vi "Panel.vi"(11 "StokePlot.lvlib:SinglePlotPanel.lvclass":refnum<class "RocketPlotPanel.lvclass">) -> ()   [LabVIEW 2021, in "RocketPlot.lvlib" / "RocketPlotPanel.lvclass"]
uses:
  RocketPlotPanel.lvclass
  RocketPlotPanel.lvclass/RocketPlotPanel.ctl
  <vilib>/Utility/miscctls.llb/LVPointTypeDef.ctl
  RocketPlot.lvlib
  TypeDefs/Plot UI references.ctl
  RocketPlotHandle/RocketPlotHandle.lvclass
  TypeDefs/plot while loop data.ctl
  <vilib>/Futures/Futures/Promise/Promise.lvclass
  TypeDefs/Save 1PLOT config.ctl
  RocketPlotHandle/SubVIs/Load config options.ctl
  TypeDefs/Plot general properties.ctl
  TypeDefs/Plot scale axis properties.ctl
  TypeDefs/plot attributes V2.ctl
  TypeDefs/plot properties V2.ctl
  TypeDefs/plot load data V2.ctl
  RocketPlotHandle/SubVIs/Load config.ctl
  SubVIs/CollapsePanel/CollapsePanel.lvclass
  SubVIs/CollapsePanel/SubVIs/collapse direction.ctl
  <vilib>/Utility/miscctls.llb/LVRangeTypeDef.ctl
  TypeDefs/RangeCache.ctl
  TypeDefs/MouseDownState.ctl
  <vilib>/Utility/miscctls.llb/LVPoint32TypeDef.ctl
  TypeDefs/RightClickCache.ctl
  TypeDefs/ZoomCache.ctl
  TypeDefs/RightClickCache PlatMod.ctl
  <vilib>/Utility/miscctls.llb/LVRectTypeDef.ctl
  TypeDefs/Slice average.ctl
  TypeDefs/ZoomCache PlatMod.ctl
  <userlib>/bjustice/TipStripOOPanel/Classes/TipPanelHandle/TipPanelHandle.lvclass
  <vilib>/IlluminatedG/IG OOPanel/OOPanel/Panel/Panel.lvclass
  SubVIs/Autocomplete popup/Autocomplete popup.lvlib
  SubVIs/Autocomplete popup/subvis/input options.ctl
  SubVIs/CollapsePanel/SubVIs/Expand.vi
  SubVIs/CollapsePanel/SubVIs/Collapse.vi
  SubVIs/CollapsePanel/SubVIs/Destroy.vi
  <vilib>/Utility/inputDevices.llb/closeKeyboard.vi
  TypeDefs/RightClickType.ctl
  TypeDefs/update plot queue data.ctl
  TypeDefs/plot updated return data.ctl
  TipTablePanel/TipTablePanel.lvclass
  <userlib>/bjustice/TipStripOOPanel/Classes/TipPanelHandle/CMD - shutdown.vi
  <userlib>/bjustice/TipStripOOPanel/Classes/TipPanelHandle/New.vi
  SubVIs/CollapsePanel/SubVIs/New.vi
  RocketPlotHandle/SubVIs/callback type.ctl
  RocketPlotHandle/SubVIs/callback data.ctl
  RocketPlotHandle/SubVIs/callback maximize data.ctl
  C:/Program Files/National Instruments/LabVIEW 2021/vi.lib/IlluminatedG/IG OOPanel/OOPanel/Panel/Panel.lvclass
  C:/Users/bjustice/Documents/GitHub/BluePlot/Source/Classes/RocketPlotPanel/RocketPlotPanel.lvclass
  C:/Program Files/National Instruments/LabVIEW 2021/user.lib/bjustice/TipStripOOPanel/Classes/TipPanel/TipPanel.lvclass
  C:/Users/bjustice/Documents/GitHub/BluePlot/Source/Classes/TipTablePanel/TipTablePanel.lvclass
  TypeDefs/Plot top row.ctl
  TypeDefs/TimeZone.ctl
  TypeDefs/AxisFocus.ctl
  SubVIs/menu/Plot menu activation submenu type v2.ctl
  TypeDefs/Plot axis.ctl
  TypeDefs/Shortcut Location.ctl
panel:
  in  "Plot Updated":T1
  in  "shutdown?":bool
  out "Location":T3
  out "DeferResize?":bool
  out "ShowPlotToolbar":bool
  in  "TimeZone":T6
  in  "Save 1PLOT (spoof)":bool
  in  "Load 1PLOT (spoof)":bool
  in  "Open Settings (spoof)":bool
  in  "Tab":enum32{"Page 1"}(tab)
  in  "x-axis name":string
  in  "Add row":bool
  in  "Time to Plot":dbl=1800.0 format="%<%H:%M:%S>t"
  in  "Title Visible?":bool
  in  "Erase Plot":bool
  in  "Open Settings":bool
  in  "Save 1PLOT":bool
  in  "Load 1PLOT":bool
  in  "x-axis not time?":bool caption="enable non-time x-axis?"
  in  "Scrollbar":i32(c297)
  in  "spoof1":T7(graph)
  in  "top array":T8[](array[typedef])
  in  "Title":string="Title"
  in  "PlotButtonsTab":enum32{"Page 1"}(tab)
  in  "Info":bool
  in  "max":bool
  in  "visible sidebar?":bool
  in  "Plot":cluster{dbl[], "Data":dbl[]}[](graph)
  out "RightAxisFocus":T9
  out "LeftAxisFocus":T9
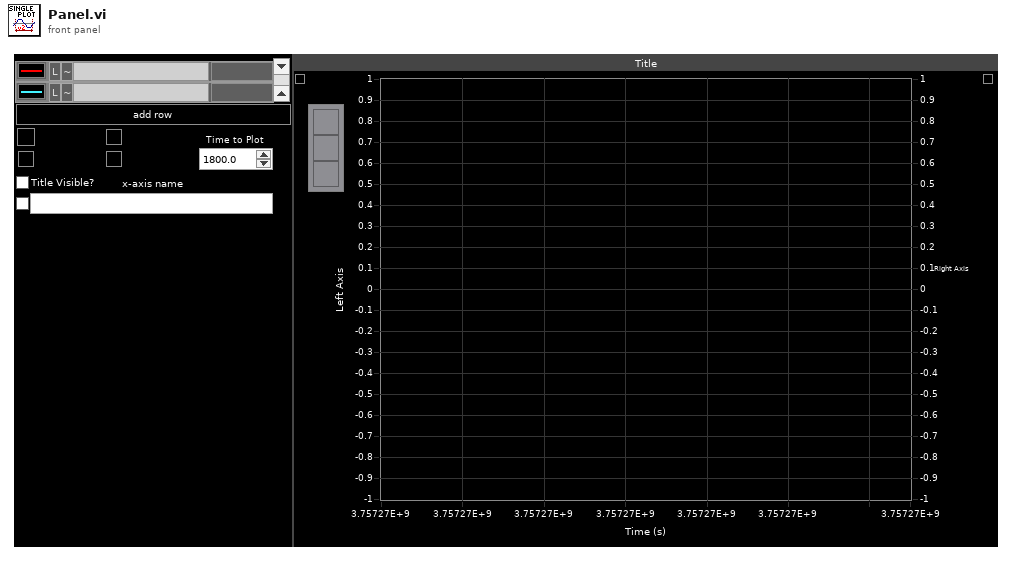
[diagram p1: front panel]
types:
  T1 = typedef "RocketPlot.lvlib/plot updated return data.ctl" = cluster{"Numerics":dbl[], "RightClickCache.slice":T2[]}
  T2 = typedef "RocketPlot.lvlib/Slice average.ctl" = cluster{"PlotIndex":i32, "Min":dbl, "Max":dbl, "Avg":dbl, "#points":u32, "Rate (Hz)":dbl, "Integral":dbl, "sigma":dbl, "CV":dbl}
  T3 = typedef "RocketPlot.lvlib/Shortcut Location.ctl" = cluster{"Location":T4, "Location.Scale":T5}
  T4 = typedef "RocketPlot.lvlib/Plot menu activation submenu type v2.ctl" = enum16{"plot area", "plot border", "markers", "scale"}
  T5 = typedef "RocketPlot.lvlib/Plot axis.ctl" = enum16{"x axis", "left axis", "right axis"}
  T6 = typedef "RocketPlot.lvlib/TimeZone.ctl" = enum16{"UTC", "Local"}
  T7 = cluster{cluster{"Time Stamp":dbl, "Data Value":dbl}[]}[]
  T8 = typedef "RocketPlot.lvlib/Plot top row.ctl" = cluster{"PID":string, "index":i32, "PID color":u32, "right axis?":bool, "Flatline?":bool, "Numeric color":u32, "Data":string, "Flat":string}
  T9 = typedef "RocketPlot.lvlib/AxisFocus.ctl" = bool
  T10 = typedef "RocketPlot.lvlib/update plot queue data.ctl" = cluster{"RightClickType":T11, "CoordsStart":T12, "CoordsEnd":T12}
  T11 = typedef "RocketPlot.lvlib/RightClickType.ctl" = enum16{"Idle", "Delta", "SliceAvg", "Identify"}
  T12 = typedef "LVPoint32TypeDef.ctl" = cluster{"Horizontal":i32, "Vertical":i32}
  T13 = typedef "CollapsePanel.lvclass/collapse direction.ctl" = enum16{"Left", "Right", "Up", "Down"}
  T14 = typedef "RocketPlot.lvlib/plot while loop data.ctl" = cluster{"TitleCollapse":refnum<class "CollapsePanel.lvclass">, "MouseDownState":T15, "RightClickCache":T16, "ZoomCache":T19, "UpdateTime":dbl, "keyboard":refnum<k1>, "visible?":bool}
  T15 = typedef "RocketPlot.lvlib/MouseDownState.ctl" = enum16{"Idle", "Pan", "Zoom", "Zoom-Post", "RightClick"}
  T16 = typedef "RocketPlot.lvlib/RightClickCache.ctl" = cluster{"Mod":T17, "CoordsStart":T12, "CoordsEnd":T12, "PlotAreaBounds":T18, "slice":T2[]}
  T17 = typedef "RocketPlot.lvlib/RightClickCache PlatMod.ctl" = cluster{"Ctrl":bool, "Shift":bool}
  T18 = typedef "LVRectTypeDef.ctl" = cluster{"Left":i16, "Top":i16, "Right":i16, "Bottom":i16}
  T19 = typedef "RocketPlot.lvlib/ZoomCache.ctl" = cluster{"SuppressedPlots":i32[], "LeftAxis":T20, "RightAxis":T20, "Mod":T22}
  T20 = typedef "RocketPlot.lvlib/RangeCache.ctl" = cluster{"NeedsRevert?":bool, "Scale Fit":u8, "Range":T21}
  T21 = typedef "LVRangeTypeDef.ctl" = cluster{"Minimum":dbl, "Maximum":dbl, "Increment":dbl, "Minor Increment":dbl, "Start":dbl}
  T22 = typedef "RocketPlot.lvlib/ZoomCache PlatMod.ctl" = cluster{"Shift":bool}
  T23 = typedef "RocketPlot.lvlib/Plot UI references.ctl" = cluster{"Title":refnum<vi>, "Title?":refnum<vi>, "Visible sidebar?":refnum<vi>, "Time to Plot":refnum<vi>, "top array":refnum<vi>, "Scrollbar":refnum<vi>, "tab ref":refnum<vi>, "Add row":refnum<vi>, "TopArray":cluster{"PID":refnum<vi>, "Numeric color":refnum<vi>, "Flat":refnum<vi>, "PID color":refnum<vi>, "Data":refnum<vi>}, "Splitter":refnum<vi>, "Front Panel":refnum<vi>, "VI":refnum<vi>, "Meta LUT":refnum<data-value>, "spoof":refnum<vi>, "BluePlotHandle":refnum<class "RocketPlotHandle.lvclass">, "PlotPane":refnum<vi>, "X Scale":refnum<vi>, "Left Scale":refnum<vi>, "Right Scale":refnum<vi>, "TimeZone":refnum<vi>, "ShowPlotToolBar":refnum<vi>, "DeferResize?":refnum<vi>, "LegendPane":refnum<vi>, "Plot":refnum<vi>, "PlotToolBar":refnum<vi>, "TB.Info":refnum<vi>, "TB.max":refnum<vi>, "X Scale.Plot Name":refnum<vi>, "X Scale.Use Plot Name?":refnum<vi>, "TipPanel":refnum<class "TipPanelHandle.lvclass">}
  T24 = typedef "RocketPlotHandle.lvclass/Init Options.ctl" = cluster{"UI visible?":bool, "Update rate (ms)":u32, "Sidebar.Visible":bool, "time to plot (init)":dbl, "time to plot (max)":dbl, "config file start path":path, "Title.Visible":bool, "Title":string, "TimeZone":T6}
  T25 = typedef "LVPointTypeDef.ctl" = cluster{"Horizontal":i16, "Vertical":i16}
  T26 = typedef "OOPanel.lvlib/Panel.lvclass/Panel Events.ctl" = cluster{"Visbility":refnum<user-event>, "Close":refnum<user-event>}
  T27 = typedef "RocketPlot.lvlib/panel mode.ctl" = enum16{"1PLOT", "MPLOT"}
  T28 = typedef "RocketPlotHandle.lvclass/callback type.ctl" = enum16{"Maximize", "ShortcutMenu"}
  T29 = typedef "RocketPlotHandle.lvclass/callback data.ctl" = cluster{"Type":T28, "data":variant, "owning subpanel":refnum<vi>}
  T30 = typedef "RocketPlot.lvlib/Save 1PLOT config.ctl" = cluster{"file extension":string, "start path":path}
  T31 = typedef "RocketPlotHandle.lvclass/Load config options.ctl" = cluster{"Load plots?":bool, "Load X-axis?":bool, "Load Y-axes?":bool, "Load General?":bool}
  T32 = typedef "RocketPlotHandle.lvclass/Load config.ctl" = cluster{"Plot config":T33, "Load options (All)":T31}
  T33 = typedef "RocketPlot.lvlib/plot load data V2.ctl" = cluster{"plots":T34[], "X-axis":T36, "Y-axes":T36[], "General":T37}
  T34 = typedef "RocketPlot.lvlib/plot properties V2.ctl" = cluster{"attributes":T35, "Numeric":dbl, "Flatline?":bool}
  T35 = typedef "RocketPlot.lvlib/plot attributes V2.ctl" = cluster{"Plot Color":u32, "Point Style":u8, "Line Style":u8, "Plot Interpolation":u8, "Line Width":u8, "Bar Plot Style":u8, "Fill To":i16, "X Scale Index":u32, "Y Scale Index":u32, "Anti-aliased":bool, "Label Format":u8, "Digital Transition Type":u8, "Digital Transition Location":u8, "Digital Line Style":u8, "Fill/Point Color":u32, "Plot Name":string, "Visible":bool}
  T36 = typedef "RocketPlot.lvlib/Plot scale axis properties.ctl" = cluster{"Name Label.Text":string, "Style":u8, "Tick Colors:Minor Tick Color":u32, "Tick Colors:Tick Color":u32, "Marker Colors:Text Color":u32, "Grid Colors:Major Color":u32, "Grid Colors:Minor Color":u32, "Mapping Mode":u8, "Flipped":bool, "Name Label.Visible":bool, "Name Label.Text Colors:Text Color":u32, "Scale Fit":u8, "Range:Maximum":dbl, "Range:Minimum":dbl, "Offset and Multiplier:Multiplier":dbl, "Offset and Multiplier:Offset":dbl, "Name Label.Font:Size":u32, "Marker.Font:Size":u32, "Uniform Marker Spacing?":bool, "Format String":string}
  T37 = typedef "RocketPlot.lvlib/Plot general properties.ctl" = cluster{"Title":string, "Time to Plot":dbl, "Title.Visible":bool, "Sidebar.Visible":bool, "Plot Area:Colors:BG Color":u32, "X Scale.Plot Name":string, "X Scale.Use Plot Name":bool}
  T38 = typedef "RocketPlotHandle.lvclass/callback maximize data.ctl" = cluster{"Maximize?":bool, "max button":refnum<vi>}
  T39 = typedef "Autocomplete popup.lvlib/input options.ctl" = cluster{"Screen Coordinates":T25, "Width":u32, "max rows":i32, "List":string[], "init value":string}
  T40 = cluster{"Color":u32, "PointStyle":u8, "LineStyle":u8, "Interp":u8, "LineWidth":u8, "BarPlotStyle":u8, "FillTo":i16, "XScaleIdx":u32, "YScaleIdx":u32, "Anti-Aliased":bool, "LabelFormat":u8, "TransitionType":u8, "TransitionLocation":u8, "DigitalLineStyle":u8}
  T41 = typedef "Plot top row.ctl" = cluster{"PID":string, "index":i32, "PID color":u32, "right axis?":bool, "Flatline?":bool, "Numeric color":u32, "Data":string, "Flat":string}
  T42 = typedef "RocketPlot.lvlib/TipTablePanel.lvclass/cell cache.ctl" = cluster{"text":string, "Color":u32, "Justification":enum16{"Left", "Center", "Right"}}
  T43 = typedef "StokePlot.lvlib/Plot QSM action.ctl" = enum16{"Get Config", "Load Config", "Set TimeToPlot", "Clear Config"}
  T44 = typedef "OOPanel.lvlib/Visibility State.ctl" = enum16{"Idle", "Closed", "Hidden", "Visible", "Subpanel", "Hidden Subpanel"}
  T45 = cluster{"Shift":bool, "Ctrl":bool, "Alt":bool, "Cmd":bool, "Opt":bool}
  T46 = typedef "eventvkey.ctl" = enum16{"ASCII", "Enter", "Return", "Shift", "Ctrl", "Alt", "Cmd", "Opt", "Caps", "NumLock", "Clear", "Break", "Up", "Down", "Left", "Right", "Insert", "Delete", "Home", "End", "PageUp", "PageDown", "Escape", "Help", "Pause", "ScrollLock", "F1", "F2", "F3", "F4", "F5", "F6", "F7", "F8", "F9", "F10", "F11", "F12", "F13", "F14", "F15", "F16", "F17", "F18", "F19", "F20", "F21", "F22", "F23", "F24", "Play", "VolumeUp", "VolumeDown", "Mute", "Two Byte Char"}
  T47 = typedef "RocketPlot.lvlib/Plot scale meta JSON.ctl" = cluster{"Type":T5, "Grid Colors:Major Color":u32, "Grid Colors:Minor Color":u32, "Style":u8, "Tick Colors:Tick Color":u32, "Tick Colors:Minor Tick Color":u32, "Format String":string, "State":T48, "AxisFocus":refnum<vi>}
  T48 = typedef "RocketPlot.lvlib/Plot scale meta state.ctl" = cluster{"Visible":bool, "Focus":bool, "Multi-Y":bool}
  T49 = typedef "TimeZone.ctl" = enum16{"UTC", "Local"}
  T50 = typedef "LVPositionTypeDef.ctl" = cluster{"Left":i32, "Top":i32}
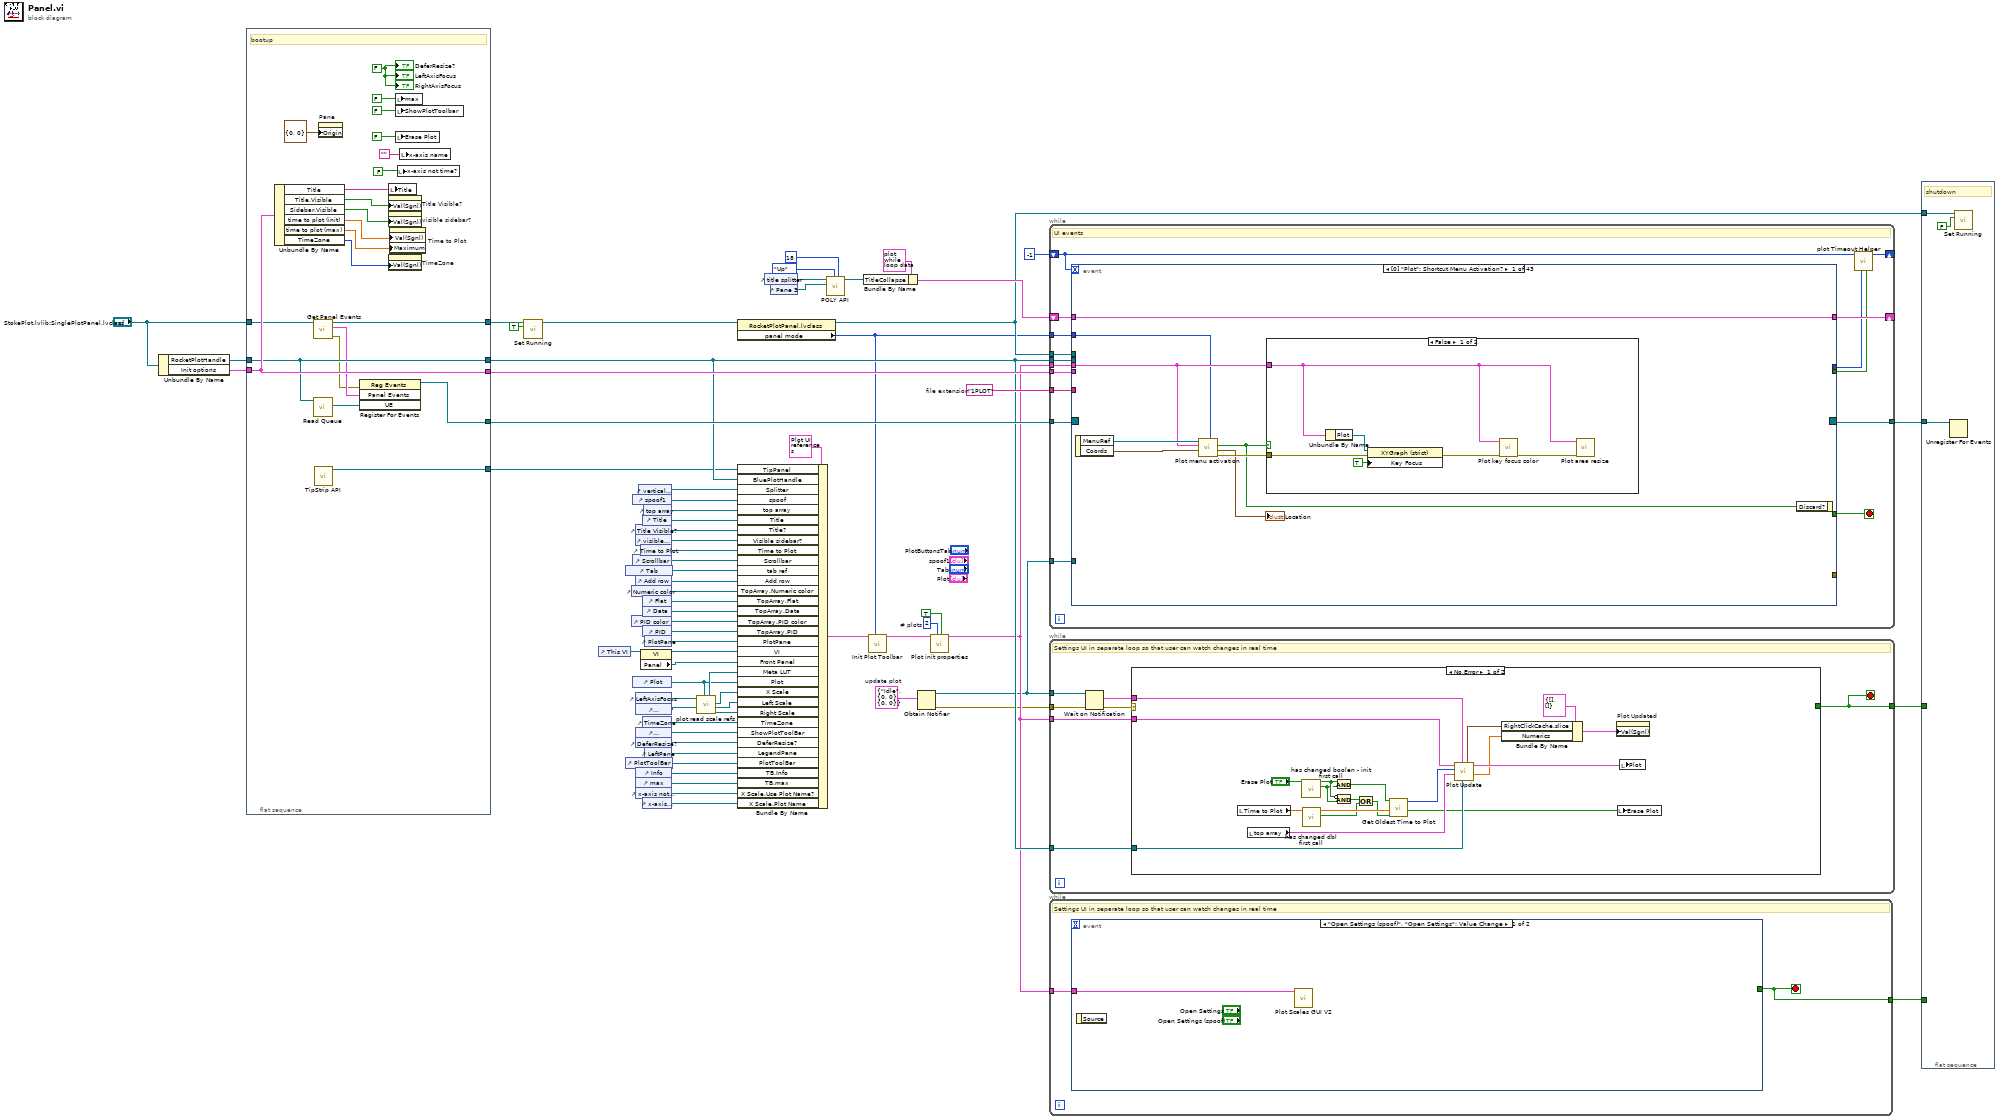
[diagram p0: block diagram]
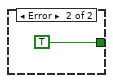
[diagram p2: hidden frame]
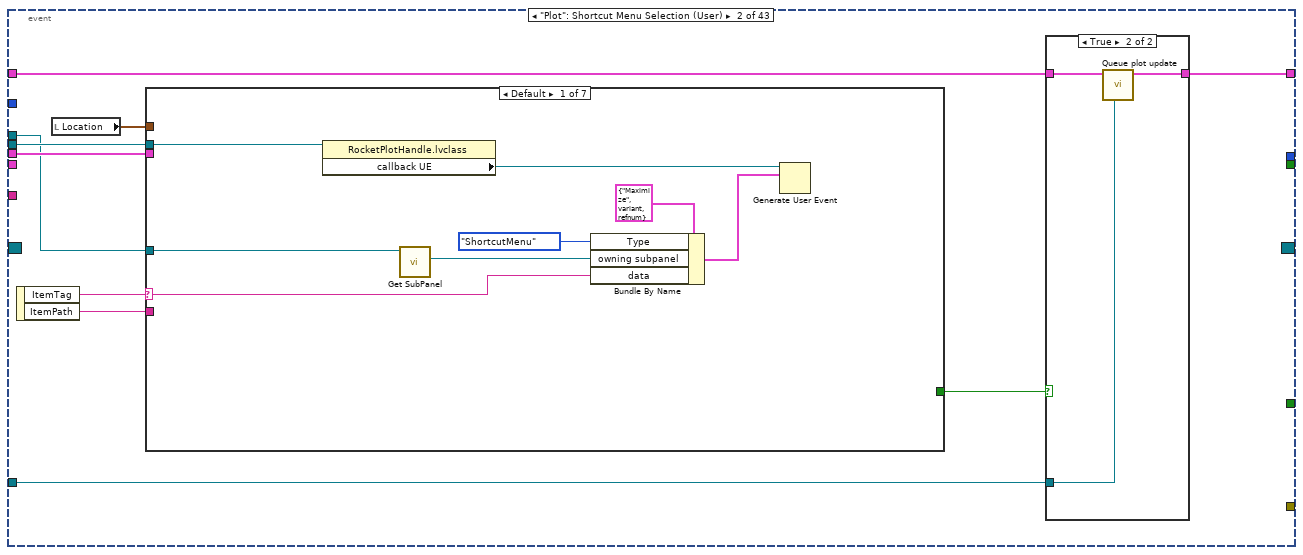
[diagram p4: hidden frame]
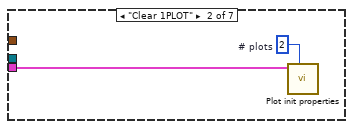
[diagram p6: hidden frame]
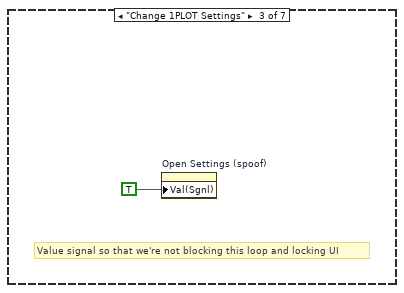
[diagram p7: hidden frame]
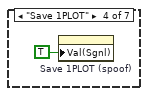
[diagram p8: hidden frame]
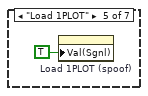
[diagram p9: hidden frame]
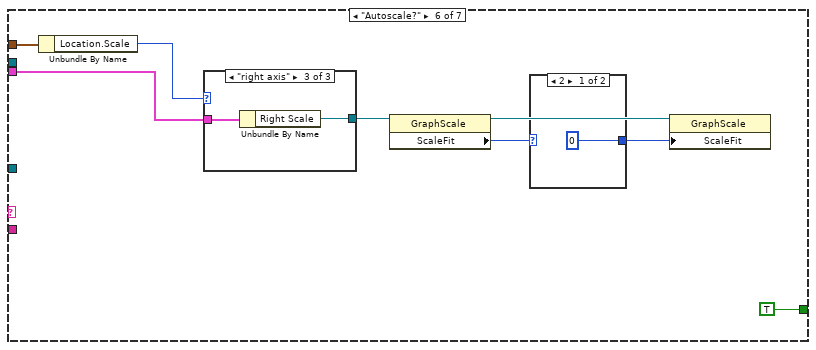
[diagram p10: hidden frame]
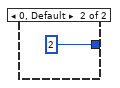
[diagram p11: hidden frame]
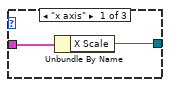
[diagram p12: hidden frame]
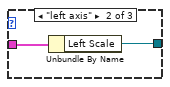
[diagram p13: hidden frame]
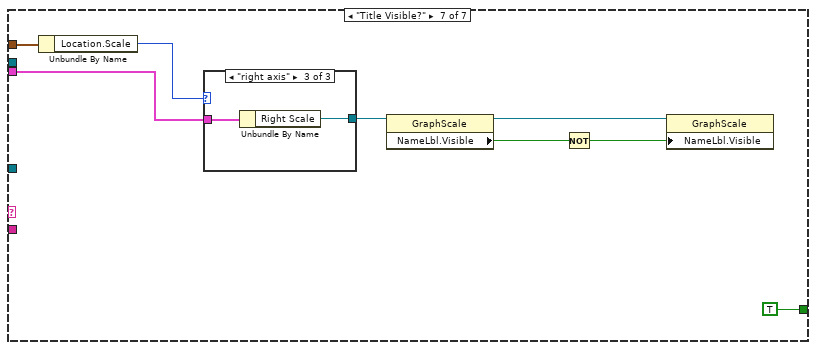
[diagram p14: hidden frame]
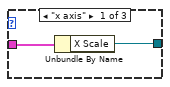
[diagram p15: hidden frame]
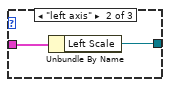
[diagram p16: hidden frame]
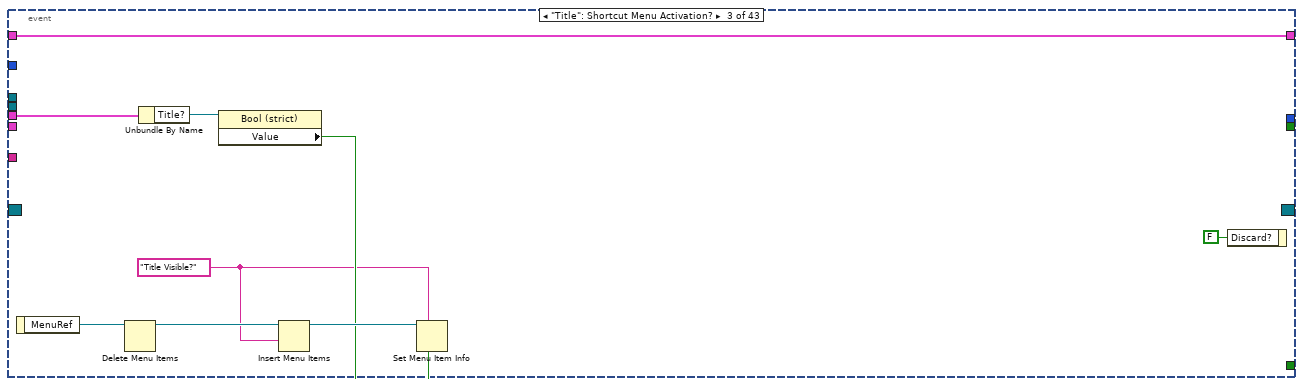
[diagram p17: hidden frame]
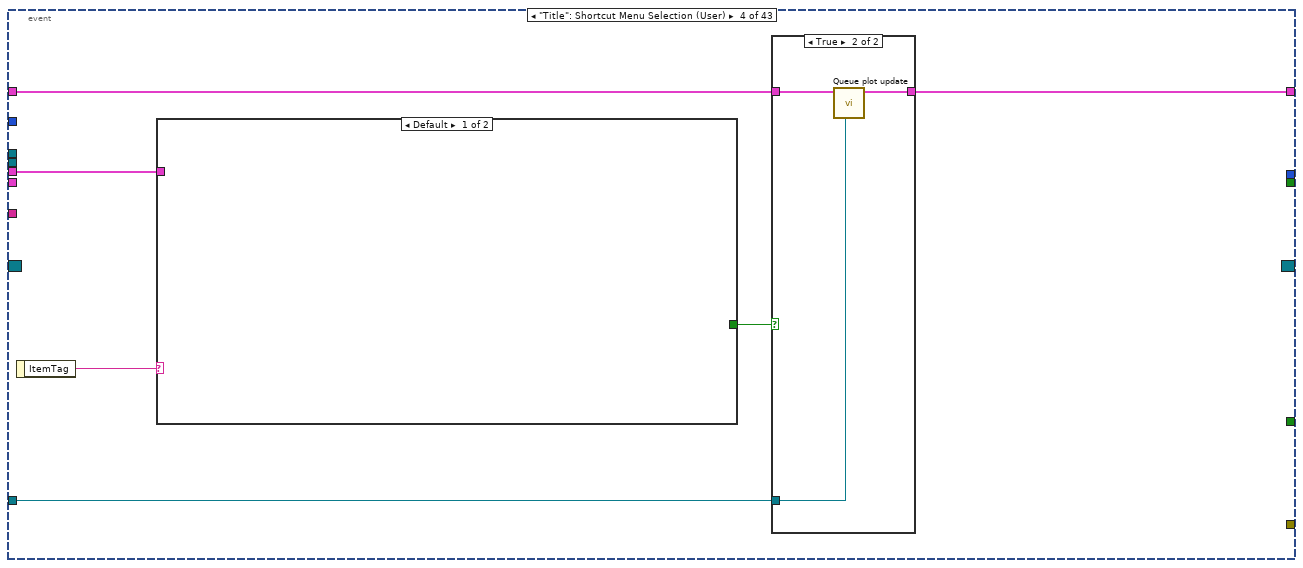
[diagram p18: hidden frame]
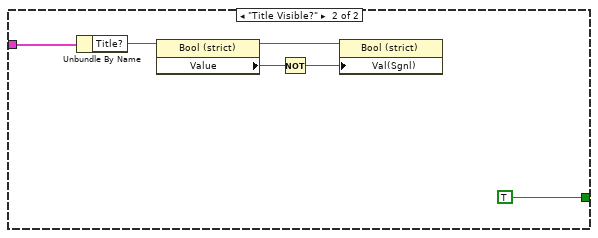
[diagram p20: hidden frame]
diagram:
  w7 = T10 {"RightClickType"=enum."Idle", "CoordsStart"={"Horizontal"=0, "Vertical"=0}, "CoordsEnd"={"Horizontal"=0, "Vertical"=0}}  # update plot
  w49 = "1PLOT"  # file extension
  w62 = 2  # # plots
  n1 = Unbundle By Name("StokePlot.lvlib:SinglePlotPanel.lvclass") -> ("RocketPlotHandle"=w17:refnum<class "RocketPlotHandle.lvclass">, "Init options"=w18:T24)
  n2 = flat-sequence {
    tunnel: [w90] -> w47
    tunnel: [w83] -> w9
    tunnel: w17 -> [w83]
    tunnel: w18 -> [w84]
    tunnel: [w84] -> w46
    tunnel: "StokePlot.lvlib:SinglePlotPanel.lvclass" -> [w76]
    tunnel: [w72] -> w15
    tunnel: [w70] -> w4
    frame #0 {
      w78 = FALSE ("DeferResize?")
      # "bootup"
      n3 = Unbundle By Name(w84) -> ("Title"=w89:string, "Title.Visible"=w88:bool, "Sidebar.Visible"=w80:bool, "time to plot (init)"=w86:dbl, "time to plot (max)"=w87:dbl, "TimeZone"=w69:T6)
      n4 = call <vilib>:"Get Panel Events.vi"("Panel in"=w76) -> ("error out"=w74:errorcluster, "Panel Events"=w75:T26, "Panel out"=w72:refnum<class "RocketPlotPanel.lvclass">)  [unwired: 8 in]
      n5 = call "Read Queue.vi"("BluePlotHandle in"=w83) -> ("UE"=w77:refnum<user-event>)  [unwired: 8 in, 2 out]
      n6 = call-poly <userlib>:"TipStrip API.vi"() -> ("TipPanelHandle out"=w70:refnum<class "TipPanelHandle.lvclass">)  [unwired: 10 in, 1 out]
      n7 = property on="Pane" class="Pane"("Origin"=T25 {"Horizontal"=0, "Vertical"=0}) -> ()  [unwired: 2 in, 2 out]
      n8 = register-events(error in=w74, w75, w77) -> (reference out=w90:refnum<event-registration>)  [unwired: 1 in, 1 out]
      n9 = local write "Title"(w89) -> ()
      n10 = property on="Title Visible?" class="Bool (strict)"("Val(Sgnl)"=w88) -> ()  [unwired: 2 in, 2 out]
      n11 = property on="visible sidebar?" class="Bool (strict)"("Val(Sgnl)"=w80) -> ()  [unwired: 2 in, 2 out]
      n12 = property on="TimeZone" class="Enum (strict)"("Val(Sgnl)"=w69) -> ()  [unwired: 2 in, 2 out]
      n13 = property on="Time to Plot" class="DigNum (strict)"("Val(Sgnl)"=w86, "Maximum"=w87) -> ()  [unwired: 2 in, 2 out]
      n14 = local write "max"(FALSE ("max")) -> ()
      n15 = local write "ShowPlotToolbar"(FALSE ("ShowCollapseButton")) -> ()
      n16 = local write "Erase Plot"(FALSE ("Clear Plots")) -> ()
      n17 = local write "x-axis not time?"(FALSE ("Value (Signaling)")) -> ()
      n18 = local write "x-axis name"("") -> ()
      "LeftAxisFocus" <- w78
      "RightAxisFocus" <- w78
      "DeferResize?" <- w78
    }
  }
  n19 = call <vilib>:"Set Running.vi"("Running"=TRUE, "Panel in"=w15) -> ("Panel out"=w3:refnum<class "RocketPlotPanel.lvclass">)  [unwired: 8 in, 1 out]
  n20 = control-ref of="This VI"() -> (w58:refnum<vi>)
  n21 = control-ref of="Tab"() -> (w63:refnum<vi>)
  n22 = control-ref of="PlotToolBar"() -> (w24:refnum<vi>)
  n23 = control-ref of="Numeric color"() -> (w53:refnum<vi>)
  n24 = control-ref of="PID color"() -> (w50:refnum<vi>)
  n25 = control-ref of="spoof1"() -> (w61:refnum<vi>)
  n26 = control-ref of="Scrollbar"() -> (w64:refnum<vi>)
  n27 = control-ref of="Plot"() -> (w26:refnum<vi>)
  n28 = control-ref of="Title Visible?"() -> (w66:refnum<vi>)
  n29 = control-ref of="visible sidebar?"() -> (w25:refnum<vi>)
  n30 = control-ref of="Add row"() -> (w59:refnum<vi>)
  n31 = control-ref of="LeftAxisFocus"() -> (w37:refnum<vi>)
  n32 = control-ref of="RightAxisFocus"() -> (w36:refnum<vi>)
  n33 = control-ref of="ShowPlotToolbar"() -> (w38:refnum<vi>)
  n34 = control-ref of="DeferResize?"() -> (w28:refnum<vi>)
  n35 = control-ref of="Info"() -> (w23:refnum<vi>)
  n36 = control-ref of="max"() -> (w22:refnum<vi>)
  n37 = control-ref of="x-axis not time?"() -> (w14:refnum<vi>)
  n38 = control-ref of="vertical splitter"() -> (w57:refnum<vi>)
  n39 = control-ref of="Time to Plot"() -> (w67:refnum<vi>)
  n40 = property class="VI"(reference=w58) -> (reference out=w55:refnum<vi>, "Panel"=w56:refnum<vi>)  [unwired: 1 in, 1 out]
  n41 = control-ref of="Title"() -> (w65:refnum<vi>)
  n42 = control-ref of="Flat"() -> (w52:refnum<vi>)
  n43 = control-ref of="Data"() -> (w51:refnum<vi>)
  n44 = control-ref of="PID"() -> (w54:refnum<vi>)
  n45 = control-ref of="TimeZone"() -> (w40:refnum<vi>)
  n46 = control-ref of="x-axis name"() -> (w11:refnum<vi>)
  n47 = control-ref of="top array"() -> (w60:refnum<vi>)
  n48 = control-ref of="PlotPane"() -> (w48:refnum<vi>)
  n49 = control-ref of="LeftPane"() -> (w27:refnum<vi>)
  n50 = call "plot read scale refs.vi"("Plot"=w26, "RightAxisFocus"=w36, "LeftAxisFocus"=w37) -> ("Right Scale"=w43:refnum<vi>, "Left Scale"=w42:refnum<vi>, "X Scale"=w41:refnum<vi>, "Meta LUT"=w39:refnum<data-value>)  [unwired: 4 in, 1 out]
  n51 = property class="RocketPlotPanel.lvclass"(reference=w3) -> (reference out=w2:refnum<class "RocketPlotPanel.lvclass">, "panel mode"=w1:T27)  [unwired: 1 in, 1 out]
  n52 = Bundle By Name(cluster=T23 {"Title"=refnum, "Title?"=refnum, "Visible sidebar?"=refnum, "Time to Plot"=refnum, "top array"=refnum, "Scrollbar"=refnum, "tab ref"=refnum, "Add row"=refnum, "TopArray"={"PID"=refnum, "Numeric color"=refnum, "Flat"=refnum, "PID color"=refnum, "Data"=refnum}, "Splitter"=refnum, "Front Panel"=refnum, "VI"=refnum, "Meta LUT"=refnum, "spoof"=refnum, "BluePlotHandle"=refnum, "PlotPane"=refnum, "X Scale"=refnum, "Left Scale"=refnum, "Right Scale"=refnum, "TimeZone"=refnum, "ShowPlotToolBar"=refnum, "DeferResize?"=refnum, "LegendPane"=refnum, "Plot"=refnum, "PlotToolBar"=refnum, "TB.Info"=refnum, "TB.max"=refnum, "X Scale.Plot Name"=refnum, "X Scale.Use Plot Name?"=refnum, "TipPanel"=refnum} ("Cluster"), "TipPanel"=w4, "BluePlotHandle"=w9, "Splitter"=w57, "spoof"=w61, "top array"=w60, "Title"=w65, "Title?"=w66, "Visible sidebar?"=w25, "Time to Plot"=w67, "Scrollbar"=w64, "tab ref"=w63, "Add row"=w59, "TopArray.Numeric color"=w53, "TopArray.Flat"=w52, "TopArray.Data"=w51, "TopArray.PID color"=w50, "TopArray.PID"=w54, "PlotPane"=w48, "VI"=w55, "Front Panel"=w56, "Meta LUT"=w39, "Plot"=w26, "X Scale"=w41, "Left Scale"=w42, "Right Scale"=w43, "TimeZone"=w40, "ShowPlotToolBar"=w38, "DeferResize?"=w28, "LegendPane"=w27, "PlotToolBar"=w24, "TB.Info"=w23, "TB.max"=w22, "X Scale.Use Plot Name?"=w14, "X Scale.Plot Name"=w11) -> (w21:T23)
  n53 = control-ref of="title splitter"() -> (w33:refnum<vi>)
  n54 = control-ref of="Pane 3"() -> (w32:refnum<vi>)
  n55 = call-poly "POLY API.vi"("ExpandSize (starting size)"=18, "CollapseDirection"=collapse_direction."Up", "Pane"=w32, "Splitter"=w33) -> ("CollapsePanel out"=w30:refnum<class "CollapsePanel.lvclass">)  [unwired: 6 in, 1 out]
  n56 = Bundle By Name(cluster=T14 {"TitleCollapse"=refnum, "MouseDownState"=enum."Idle", "RightClickCache"={"Mod"={"Ctrl"=FALSE, "Shift"=FALSE}, "CoordsStart"={"Horizontal"=0, "Vertical"=0}, "CoordsEnd"={"Horizontal"=0, "Vertical"=0}, "PlotAreaBounds"={"Left"=10, "Top"=10, "Right"=0, "Bottom"=0}, "slice"=[]}, "ZoomCache"={"SuppressedPlots"=[], "LeftAxis"={"NeedsRevert?"=FALSE, "Scale Fit"=0, "Range"={"Minimum"=0.0, "Maximum"=0.0, "Increment"=0.0, "Minor Increment"=0.0, "Start"=0.0}}, "RightAxis"={"NeedsRevert?"=FALSE, "Scale Fit"=0, "Range"={"Minimum"=0.0, "Maximum"=0.0, "Increment"=0.0, "Minor Increment"=0.0, "Start"=0.0}}, "Mod"={"Shift"=FALSE}}, "UpdateTime"=0.0, "keyboard"=refnum, "visible?"=FALSE} ("loop data"), "TitleCollapse"=w30) -> (w29:T14)
  n57 = call "Init Plot Toolbar.vi"("panel mode"=w1, "Refs"=w21) -> ("Refs (dup)"=w20:T23)  [unwired: 8 in, 1 out]
  n58 = Obtain Notifier(notification data type=w7) -> (notifier out=w6:refnum<notifier>, error out=w5:errorcluster)  [unwired: 3 in, 1 out]
  n59 = call "Plot init properties.vi"("First call? (init)"=TRUE, "# plots"=w62, "Refs"=w20) -> ("Refs (dup)"=w8:T23)  [unwired: 7 in, 1 out]
  n60 = while {
    tunnel: w8 -> [w106]
    tunnel: w9 -> [w105]
    tunnel: w46 -> [w104]
    tunnel: w49 -> [w103]
    tunnel: w47 -> [w102]
    shift-right: [w97] -> _
    shift-left: -1 ("Timeout") -> [w96]
    tunnel: [w100] -> w45
    shift-right: [w98] -> _
    shift-left: w29 -> [w99]
    tunnel: w6 -> [w93]
    tunnel: w2 -> [w92]
    tunnel: w1 -> [w91]
    stop <- w101 stop-if-true
    # "UI events"
    n61 = event shown="[0] \"Plot\": Shortcut Menu Activation?" {
      selector: w102 -> [_ _ _ _ _ _ _ _ _ _ _ _ _ _ _ _ _ _ _ _ _ _ _ _ _ _ _ _ _ _ _ _ _ _ _ _ _ _ _ _ _ _ _]
      dyn-events: [_ _ _ _ _ _ _ _ _ _ _ _ _ _ _ _ _ _ _ _ _ _ _ _ _ _ _ _ _ _ _ _ _ _ _ _ _ _ _ _ _ _ _] -> w100
      timeout: w96 -> [_ _ _ _ _ _ _ _ _ _ _ _ _ _ _ _ _ _ _ _ _ _ _ _ _ _ _ _ _ _ _ _ _ _ _ _ _ _ _ _ _ _ _]
      tunnel: [_ _ _ _ w209 w218 _ w230 w239 w252 w265 w282 _ _ _ w305 _ _ w320 _ _ _ _ _ _ _ _ _ _ _ _ _ _ _ _ _ _ _ _ _ _ _ _] -> _
      tunnel: w106 -> [w112 w127 w183 w191 w210 w211 _ w229 w238 w251 _ w277 w291 w299 _ w306 w311 w316 w324 w329 _ w377 w386 w404 w424 w439 w468 w484 w492 w505 w529 w548 w554 w560 w564 w579 w584 w595 w610 w630 w657 w670 w674]
      tunnel: w105 -> [_ w129 _ _ _ _ _ _ _ _ _ _ _ _ w303 _ _ _ _ w328 _ w372 _ _ _ _ _ _ _ _ _ _ _ _ _ w569 _ _ _ w631 w654 _ _]
      tunnel: w104 -> [_ _ _ _ w207 w215 _ _ _ _ _ _ _ _ _ _ _ _ _ w325 w365 _ w389 _ w423 _ w473 w481 _ w499 w524 _ _ _ _ _ _ _ _ _ _ _ _]
      tunnel: w103 -> [_ _ _ _ w204 w213 _ _ _ _ _ _ _ _ _ _ _ _ _ _ _ _ _ _ _ _ _ _ _ _ _ _ _ _ _ _ _ _ _ _ _ _ _]
      tunnel: [_ _ _ _ _ _ _ _ _ _ _ _ _ _ _ _ _ _ _ _ w366 _ w387 _ w421 _ _ w482 _ _ _ _ _ _ _ _ _ _ _ _ _ _ _] -> w95
      tunnel: [_ _ _ _ _ _ _ _ _ _ _ _ _ _ _ _ _ _ _ _ w367 _ w388 _ w422 _ _ w483 _ _ _ _ _ _ _ _ _ _ _ _ _ _ _] -> w94
      tunnel: [_ _ _ _ _ _ _ _ _ _ _ _ _ _ _ _ _ _ _ _ _ w376 _ _ _ _ _ _ _ _ _ _ _ _ _ _ _ _ _ _ _ _ _] -> w101
      tunnel: w99 -> [w113 w124 w178 w189 w203 w212 w224 w226 w237 w250 w264 w283 w292 w300 w301 w304 w309 w314 w323 w327 w369 w378 w391 w407 w425 w441 w470 w485 w491 w504 w528 w547 w558 w562 w567 w580 w590 w596 w599 w632 w655 w669 w673]
      tunnel: [w113 w123 w178 w188 w203 w212 w224 w226 w237 w250 w263 w283 w292 w300 w301 w304 w309 w314 w323 w326 w368 w378 w384 w408 w420 w441 w466 w479 w487 w494 w519 w542 w558 w562 w567 w580 w590 w596 w598 w632 w655 w669 w673] -> w98
      tunnel: w93 -> [_ w122 _ w187 _ _ _ _ _ _ _ _ _ _ _ _ _ _ _ _ _ w375 w383 _ _ _ w465 w478 w486 w493 w518 w540 _ _ _ _ _ _ w597 _ _ _ _]
      tunnel: w92 -> [_ w121 _ _ _ _ _ _ _ _ _ _ _ _ _ _ _ _ _ _ _ _ _ _ _ _ _ _ _ _ _ _ _ _ _ w570 _ _ _ _ _ _ _]
      tunnel: w91 -> [w107 _ _ _ _ _ _ _ _ _ _ _ _ _ _ _ _ _ _ _ _ _ _ _ _ _ _ _ _ _ _ _ _ _ _ _ _ _ _ _ _ _ _]
      event "Plot": Shortcut Menu Activation? {
        n62 = event-data() -> ("MenuRef"=w114:refnum<k9>, "Coords"=w111:T12)  [unwired: 1 in]
        n63 = call "Plot menu activation.vi"("panel mode"=w107, "Coords"=w111, "Refs"=w112, "MenuRef"=w114) -> ("error out"=w110:errorcluster, "Location"=→"Location":T3, "Discard?"=w108:bool)  [unwired: 4 in, 1 out]
        n64 = case shown="False" w108 {
          tunnel: w112 -> [w120 _]
          tunnel: w110 -> [w118 _]
          frame False {
            n65 = Unbundle By Name(w120) -> ("Plot"=w117:refnum<vi>)
            n66 = property class="XYGraph (strict)"(reference=w117, error in=w118, "Key Focus"=TRUE) -> (error out=w115:errorcluster)  [unwired: 1 out]
            n67 = call "Plot key focus color.vi"("error in (no error)"=w115, "Refs"=w120) -> ("error out"=w116:errorcluster)  [unwired: 9 in]
            n68 = call "Plot area resize.vi"("error in (no error)"=w116, "Refs"=w120) -> ()  [unwired: 9 in, 1 out]
          }
          frame True {
          }
        }
        n69 = event-data("Discard?"=w108) -> ()  [unwired: 1 in, 1 out]
      }
      event "Plot": Shortcut Menu Selection (User) {
        n70 = event-data() -> ("ItemTag"=w130:string, "ItemPath"=w128:string)  [unwired: 1 in]
        n71 = local read "Location"() -> (w126:T3)
        n72 = case shown="Default" w130 {
          selector: w130 -> [w137 _ _ _ _ _ _]
          tunnel: w129 -> [w136 _ _ _ _ _ _]
          tunnel: w128 -> [_ _ _ _ _ _ _]
          tunnel: w127 -> [_ w143 _ _ _ w153 w169]
          tunnel: w126 -> [_ _ _ _ _ w154 w170]
          tunnel: [_ _ _ _ _ TRUE TRUE] -> w125
          tunnel: w121 -> [w135 _ _ _ _ _ _]
          frame Default {
            n73 = property class="RocketPlotHandle.lvclass"(reference=w136) -> ("callback UE"=w138:refnum<user-event>)  [unwired: 1 in, 2 out]
            n74 = call <vilib>:"Get SubPanel.vi"("Panel in"=w135) -> ("SubPanel"=w139:refnum<vi>)  [unwired: 8 in, 2 out]
            n75 = Bundle By Name(cluster=T29 {"Type"=enum."Maximize", "data"=variant(string ""), "owning subpanel"=refnum} ("event data"), "Type"=callback_type."ShortcutMenu", "owning subpanel"=w139, "data"=w137) -> (w141:T29)
            n76 = Generate User Event(user event=w138, event data cluster=w141) -> ()  [unwired: 2 in, 2 out]
          }
          frame "Clear 1PLOT" {
            w144 = 2  # # plots
            n77 = call "Plot init properties.vi"("# plots"=w144, "Refs"=w143) -> ()  [unwired: 8 in, 2 out]
          }
          frame "Change 1PLOT Settings" {
            # "Value signal so that we're not blocking this loop and locking UI"
            n78 = property on="Open Settings (spoof)" class="Bool (strict)"("Val(Sgnl)"=TRUE ("Value (Signaling)")) -> ()  [unwired: 2 in, 2 out]
          }
          frame "Save 1PLOT" {
            n79 = property on="Save 1PLOT (spoof)" class="Bool (strict)"("Val(Sgnl)"=TRUE ("Value (Signaling)")) -> ()  [unwired: 2 in, 2 out]
          }
          frame "Load 1PLOT" {
            n80 = property on="Load 1PLOT (spoof)" class="Bool (strict)"("Val(Sgnl)"=TRUE ("Value (Signaling)")) -> ()  [unwired: 2 in, 2 out]
          }
          frame "Autoscale?" {
            n81 = Unbundle By Name(w154) -> ("Location.Scale"=w152:T5)
            n82 = case shown="\"right axis\"" w152 {
              tunnel: w153 -> [w159 w161 w163]
              tunnel: [w158 w160 w162] -> w155
              frame "x axis" {
                n83 = Unbundle By Name(w159) -> ("X Scale"=w158:refnum<vi>)
              }
              frame "left axis" {
                n84 = Unbundle By Name(w161) -> ("Left Scale"=w160:refnum<vi>)
              }
              frame "right axis" {
                n85 = Unbundle By Name(w163) -> ("Right Scale"=w162:refnum<vi>)
              }
            }
            n86 = property class="GraphScale"(reference=w155) -> (reference out=w151:refnum<vi>, "ScaleFit"=w150:u8)  [unwired: 1 in, 1 out]
            n87 = case shown="2" w150 {
              tunnel: [u8 0 ("Scale Fit") u8 2 ("Scale Fit")] -> w149
              frame 2 {
              }
              frame 0, Default {
              }
            }
            n88 = property class="GraphScale"(reference=w151, "ScaleFit"=w149) -> ()  [unwired: 1 in, 2 out]
          }
          frame "Title Visible?" {
            n89 = Unbundle By Name(w170) -> ("Location.Scale"=w168:T5)
            n90 = case shown="\"right axis\"" w168 {
              tunnel: w169 -> [w173 w175 w177]
              tunnel: [w172 w174 w176] -> w171
              frame "x axis" {
                n91 = Unbundle By Name(w173) -> ("X Scale"=w172:refnum<vi>)
              }
              frame "left axis" {
                n92 = Unbundle By Name(w175) -> ("Left Scale"=w174:refnum<vi>)
              }
              frame "right axis" {
                n93 = Unbundle By Name(w177) -> ("Right Scale"=w176:refnum<vi>)
              }
            }
            n94 = property class="GraphScale"(reference=w171) -> (reference out=w167:refnum<vi>, "NameLbl.Visible"=w166:bool)  [unwired: 1 in, 1 out]
            n95 = Not(x=w166) -> (.not. x?=w165:bool)
            n96 = property class="GraphScale"(reference=w167, "NameLbl.Visible"=w165) -> ()  [unwired: 1 in, 2 out]
          }
        }
        n97 = case shown="True" w125 {
          tunnel: w124 -> [w131 w134]
          tunnel: [w131 w133] -> w123
          tunnel: w122 -> [_ w132]
          frame False {
          }
          frame True {
            n98 = call "Queue plot update.vi"("update plot notifier"=w132, "loop data in"=w134) -> ("loop data out"=w133:T14)  [unwired: 9 in]
          }
        }
      }
      event "Title": Shortcut Menu Activation? {
        w180 = "Title Visible?"
        n99 = event-data() -> ("MenuRef"=w186:refnum<k9>)  [unwired: 1 in]
        n100 = Delete Menu Items(9:w186) -> (3:w185:refnum<k9>)  [unwired: 3 in, 1 out]
        n101 = Unbundle By Name(w183) -> ("Title?"=w184:refnum<vi>)
        n102 = property class="Bool (strict)"(reference=w184) -> ("Value"=w181:bool)  [unwired: 1 in, 2 out]
        n103 = Insert Menu Items(7:w180, 9:w185) -> (3:w182:refnum<k9>)  [unwired: 4 in, 2 out]
        n104 = Set Menu Item Info(6:w181, 7:w180, 11:w182) -> ()  [unwired: 4 in, 2 out]
        n105 = event-data("Discard?"=FALSE) -> ()  [unwired: 1 in, 1 out]
      }
      event "Title": Shortcut Menu Selection (User) {
        n106 = event-data() -> ("ItemTag"=w192:string)  [unwired: 1 in]
        n107 = case shown="Default" w192 {
          tunnel: w191 -> [_ w201]
          tunnel: [_ TRUE] -> w190
          frame Default {
          }
          frame "Title Visible?" {
            n108 = Unbundle By Name(w201) -> ("Title?"=w202:refnum<vi>)
            n109 = property class="Bool (strict)"(reference=w202) -> (reference out=w199:refnum<vi>, "Value"=w200:bool)  [unwired: 1 in, 1 out]
            n110 = Not(x=w200) -> (.not. x?=w198:bool)
            n111 = property class="Bool (strict)"(reference=w199, "Val(Sgnl)"=w198) -> ()  [unwired: 1 in, 2 out]
          }
        }
        n112 = case shown="True" w190 {
          tunnel: w189 -> [w193 w196]
          tunnel: [w193 w195] -> w188
          tunnel: w187 -> [_ w194]
          frame False {
          }
          frame True {
            n113 = call "Queue plot update.vi"("update plot notifier"=w194, "loop data in"=w196) -> ("loop data out"=w195:T14)  [unwired: 9 in]
          }
        }
      }
      event "Save 1PLOT", "Save 1PLOT (spoof)": Value Change {
        n114 = event-data() -> ()  [unwired: 1 in, 1 out]
        n115 = Unbundle By Name(w207) -> ("config file start path"=w206:path)
        n116 = Bundle By Name(cluster=T30 {"file extension"="", "start path"=path ""} ("Config Ops"), "start path"=w206, "file extension"=w204) -> (w205:T30)
        n117 = call "Save 1PLOT.vi"("Refs"=w210, "Config Ops"=w205) -> ("error out"=w209:errorcluster)  [unwired: 9 in]
      }
      event "Load 1PLOT", "Load 1PLOT (spoof)": Value Change {
        n118 = event-data() -> ()  [unwired: 1 in, 1 out]
        n119 = Unbundle By Name(w215) -> ("config file start path"=w217:path)
        n120 = Bundle By Name(cluster=T30 {"file extension"="", "start path"=path ""} ("Config Ops"), "start path"=w217, "file extension"=w213) -> (w214:T30)
        n121 = call "Load 1PLOT.vi"("Config Ops"=w214) -> ("error out"=w218:errorcluster, "Valid load?"=w219:bool, "Plot Config"=w220:T33)  [unwired: 8 in]
        n122 = case shown="True" w219 {
          tunnel: w220 -> [_ w222]
          tunnel: w211 -> [_ w223]
          frame False {
          }
          frame True {
            n123 = call "Plot load reader V2.vi"("Load options (All)"=T31 {"Load plots?"=TRUE, "Load X-axis?"=TRUE, "Load Y-axes?"=TRUE, "Load General?"=TRUE}, "Plot config"=w222, "Refs"=w223) -> ()  [unwired: 8 in, 1 out]
          }
        }
      }
      event "spoof1": Shortcut Menu Selection? (App) {
        # "Don't allow this --> user right click on spoof legend outside attribute box"
        n124 = event-data() -> ()  [unwired: 1 in, 1 out]
        n125 = event-data("Discard?"=FALSE) -> ()  [unwired: 1 in, 1 out]
      }
      event "Scrollbar": Value Change {
        n126 = event-data() -> ()  [unwired: 1 in, 1 out]
        n127 = Unbundle By Name(w229) -> ("spoof"=w227:refnum<vi>, "top array"=w228:refnum<vi>)
        n128 = Build Array("Scrollbar") -> (w236:i32[])
        n129 = property class="Arr (strict)"(reference=w228, "Index Values"=w236) -> (error out=w231:errorcluster)  [unwired: 1 in, 1 out]
        n130 = property class="XYGraph"(reference=w227, "LegScrollPos"="Scrollbar") -> (reference out=w235:refnum<vi>, error out=w234:errorcluster)  [unwired: 1 in]
        n131 = call "Plot Legend NumRows.vi"("error in (no error)"=w234, "XY graph ref"=w235) -> ("error out"=w232:errorcluster)  [unwired: 8 in, 1 out]
        n132 = Merge Errors(w232, w231) -> (w230:errorcluster)
      }
      event "spoof1": Plot Attribute Change {
        n133 = event-data() -> ("PlotIdx"=w249:i32, "OldAttrib"=w248:T40, "NewAttrib"=w247:T40, "PlotRef"=w246:refnum<vi>)  [unwired: 1 in]
        n134 = Unbundle By Name(w238) -> ("Plot"=w244:refnum<vi>, "top array"=w243:refnum<vi>)
        n135 = call "Plot attribute value change event.vi"("Plot ref (target)"=w244, "top array"=w243, "PlotRef (event source)"=w246, "NewAttrib"=w247, "OldAttrib"=w248, "PlotIdx (target)"=w249) -> ("error out"=w242:errorcluster)  [unwired: 5 in]
        n136 = property class="Arr (strict)"(reference=w243, error in=w242) -> (error out=w241:errorcluster, "Value"=w245:T41[])  [unwired: 1 out]
        n137 = call "Plot Y-axis visibility.vi"("error in (no error)"=w241, "top array"=w245, "Refs"=w238) -> ("error out"=w240:errorcluster)  [unwired: 8 in]
        n138 = call "Plot area resize.vi"("error in (no error)"=w240, "Refs"=w238) -> ("error out"=w239:errorcluster)  [unwired: 9 in]
      }
      event "Plot": Plot Attribute Change {
        n139 = event-data() -> ("PlotIdx"=w261:i32, "OldAttrib"=w259:T40, "NewAttrib"=w260:T40, "PlotRef"=w262:refnum<vi>)  [unwired: 1 in]
        n140 = Unbundle By Name(w251) -> ("spoof"=w257:refnum<vi>, "top array"=w256:refnum<vi>)
        n141 = call "Plot attribute value change event.vi"("Plot ref (target)"=w257, "top array"=w256, "PlotRef (event source)"=w262, "NewAttrib"=w260, "OldAttrib"=w259, "PlotIdx (target)"=w261) -> ("error out"=w255:errorcluster)  [unwired: 5 in]
        n142 = property class="Arr (strict)"(reference=w256, error in=w255) -> (error out=w254:errorcluster, "Value"=w258:T41[])  [unwired: 1 out]
        n143 = call "Plot Y-axis visibility.vi"("error in (no error)"=w254, "top array"=w258, "Refs"=w251) -> ("error out"=w253:errorcluster)  [unwired: 8 in]
        n144 = call "Plot area resize.vi"("error in (no error)"=w253, "Refs"=w251) -> ("error out"=w252:errorcluster)  [unwired: 9 in]
      }
      event "Title Visible?": Value Change {
        n145 = event-data() -> ("NewVal"=w266:bool)  [unwired: 1 in]
        n146 = in-place {
          in-place-border: w266 -> [w270]
          in-place-border: [w269] -> w265
          n147 = in-place-cluster #1(w264) -> ("TitleCollapse"=w268:refnum<class "CollapsePanel.lvclass">)
          n148 = case shown="True" w270 {
            tunnel: w268 -> [w272 w276]
            tunnel: [w273 w275] -> w269
            tunnel: [w271 w274] -> w267
            frame False {
              n149 = call-poly "POLY API.vi"("CollapsePanel in"=w272) -> ("error out"=w273:errorcluster, "CollapsePanel out"=w271:refnum<class "CollapsePanel.lvclass">)  [unwired: 9 in]
            }
            frame True {
              n150 = call-poly "POLY API.vi"("CollapsePanel in"=w276) -> ("error out"=w275:errorcluster, "CollapsePanel out"=w274:refnum<class "CollapsePanel.lvclass">)  [unwired: 9 in]
            }
          }
          n151 = in-place-cluster #1("TitleCollapse"=w267) -> (w263:T14)
        }
      }
      event "visible sidebar?": Value Change {
        n152 = event-data() -> ("NewVal"=w280:bool)  [unwired: 1 in]
        n153 = Unbundle By Name(w277) -> ("ShowPlotToolBar"=w281:refnum<vi>)
        n154 = call "Plot resize horizontal.vi"("Refs"=w277) -> ("error out"=w282:errorcluster)  [unwired: 10 in]
        n155 = Unbundle By Name(w277) -> ("Plot"=w279:refnum<vi>)
        n156 = case shown="True" w280 {
          tunnel: w281 -> [_ w285]
          frame False {
          }
          frame True {
            n157 = property class="Bool (strict)"(reference=w285, "Value"=FALSE ("Visible")) -> ()  [unwired: 1 in, 2 out]
          }
        }
        n158 = property class="XYGraph (strict)"(reference=w279, "Key Focus"=TRUE) -> ()  [unwired: 1 in, 2 out]
      }
      event "visible sidebar?": Mouse Move {
        n159 = event-data() -> ("CtlRef"=w296:refnum<vi>)  [unwired: 1 in]
        n160 = property class="Bool (strict)"(reference=w296) -> ("Value"=w295:bool)  [unwired: 1 in, 2 out]
        n161 = Select(t="Click to Expand Sidebar  <F10>", s=w295, f="Click to Collapse Sidebar  <F10>") -> (s? t:f=w290:string)
        n162 = call "new cell.vi"("String"=w290) -> ("cell"=w289:T42)  [unwired: 10 in]
        n163 = Build Array(w289) -> (w297:T42[])
        n164 = Build Array(w297) -> (w286:T42[][])
        n165 = Unbundle By Name(w291) -> ("TipPanel"=w288:refnum<class "TipPanelHandle.lvclass">)
        n166 = call "New TipTable.vi"("show.cells"=w286) -> ("TipTablePanel out"=w287:refnum<class "TipTablePanel.lvclass">)  [unwired: 9 in, 1 out]
        n167 = call <userlib>:"CMD - show panel.vi"("TipPanel"=w287, "TipPanelHandle"=w288) -> ()  [unwired: 8 in, 2 out]
      }
      event "visible sidebar?": Mouse Leave {
        n168 = event-data() -> ()  [unwired: 1 in, 4 out]
        n169 = Unbundle By Name(w299) -> ("TipPanel"=w298:refnum<class "TipPanelHandle.lvclass">)
        n170 = call <userlib>:"CMD - hide.vi"("TipPanelHandle"=w298) -> ()  [unwired: 9 in, 2 out]
      }
      event "Time to Plot": Value Change {
        n171 = event-data() -> ()  [unwired: 1 in, 1 out]
        n172 = call-dynamic "Callback - Subscribed time to plot.vi"("time to plot (s)"="Time to Plot", "BluePlotHandle in"=w303) -> ()  [unwired: 8 in, 2 out]
      }
      event Pane Size {
        n173 = event-data() -> ()  [unwired: 1 in, 1 out]
        n174 = call "Plot resize vertical.vi"("Refs"=w306) -> ("error out"=w308:errorcluster)  [unwired: 8 in, 2 out]
        n175 = call "Plot resize horizontal.vi"("error in (no error)"=w308, "Refs"=w306) -> ("error out"=w307:errorcluster)  [unwired: 9 in]
        n176 = call "Plot area resize.vi"("error in (no error)"=w307, "Refs"=w306) -> ("error out"=w305:errorcluster)  [unwired: 9 in]
      }
      event Mouse Enter {
        n177 = event-data() -> ()  [unwired: 1 in, 1 out]
        n178 = Unbundle By Name(w311) -> ("ShowPlotToolBar"=w313:refnum<vi>)
        n179 = disable-structure shown="Disabled" {
          frame Disabled {
          }
          frame Enabled {
          }
        }
        n180 = property class="Bool (strict)"(reference=w313, "Value"=TRUE) -> (error out=w310:errorcluster)  [unwired: 1 in, 1 out]
        n181 = call "Plot area resize.vi"("error in (no error)"=w310, "Refs"=w311) -> ()  [unwired: 9 in, 1 out]
      }
      event Mouse Leave {
        n182 = event-data() -> ()  [unwired: 1 in, 1 out]
        n183 = Unbundle By Name(w316) -> ("ShowPlotToolBar"=w318:refnum<vi>)
        n184 = property class="Bool (strict)"(reference=w318, "Value"=FALSE) -> (error out=w315:errorcluster)  [unwired: 1 in, 1 out]
        n185 = call "Plot area resize.vi"("error in (no error)"=w315, "Refs"=w316) -> ()  [unwired: 9 in, 1 out]
      }
      event Value Change {
        n186 = event-data() -> ("NewVal"=w319:T6)  [unwired: 1 in]
        n187 = Unbundle By Name(w324) -> ("Meta LUT"=w322:refnum<data-value>, "X Scale"=w321:refnum<vi>)
        n188 = call "Plot axes format string.vi"("TimeZone"=w319, "Scale reference"=w321, "Meta LUT"=w322) -> ("error out"=w320:errorcluster)  [unwired: 7 in, 1 out]
      }
      event User Event {
        n189 = event-data() -> ("action"=w331:T43, "data"=w330:variant)  [unwired: 1 in]
        n190 = case shown="\"Get Config\"" w331 {
          tunnel: w330 -> [w334 w348 _ w360]
          tunnel: w329 -> [w333 w346 w356 _]
          tunnel: w328 -> [_ _ _ _]
          tunnel: w327 -> [w332 w347 w358 w359]
          tunnel: [w332 w347 w358 w359] -> w326
          tunnel: w325 -> [_ _ _ _]
          frame "Get Config" {
            n191 = Variant To Data(type=refnum<class "Promise.lvclass"> refnum ("Promise out"), Variant=w334) -> (data=w337:refnum<class "Promise.lvclass">, error out=w336:errorcluster)  [unwired: 1 in]
            n192 = case shown="No Error" w336 {
              tunnel: w333 -> [w341 _]
              tunnel: w337 -> [w340 _]
              frame No Error {
                n193 = call "Plot Load maker V2.vi"("Refs"=w341) -> ("error out"=w338:errorcluster, "Plot config"=w339:T33)  [unwired: 9 in]
                n194 = case shown="No Error" w338 {
                  selector: w338 -> [_ w344]
                  tunnel: w340 -> [w343 w345]
                  tunnel: w339 -> [w342 _]
                  frame No Error {
                    n195 = call <vilib>:"Resolve with Result.vi"("Result"=w342, "Promise in"=w343) -> ()  [unwired: 9 in, 1 out]
                  }
                  frame Error {
                    n196 = call <vilib>:"Resolve with Error.vi"("Result"=w344, "Promise in"=w345) -> ()  [unwired: 9 in, 1 out]
                  }
                }
              }
              frame Error {
              }
            }
          }
          frame "Load Config" {
            n197 = Variant To Data(type=T32 {"Plot config"={"plots"=[], "X-axis"={"Name Label.Text"="", "Style"=0, "Tick Colors:Minor Tick Color"=0, "Tick Colors:Tick Color"=0, "Marker Colors:Text Color"=0, "Grid Colors:Major Color"=0, "Grid Colors:Minor Color"=0, "Mapping Mode"=0, "Flipped"=FALSE, "Name Label.Visible"=FALSE, "Name Label.Text Colors:Text Color"=0, "Scale Fit"=0, "Range:Maximum"=0.0, "Range:Minimum"=0.0, "Offset and Multiplier:Multiplier"=0.0, "Offset and Multiplier:Offset"=0.0, "Name Label.Font:Size"=0, "Marker.Font:Size"=0, "Uniform Marker Spacing?"=TRUE, "Format String"=""}, "Y-axes"=[], "General"={"Title"="", "Time to Plot"=1800.0, "Title.Visible"=FALSE, "Sidebar.Visible"=FALSE, "Plot Area:Colors:BG Color"=0, "X Scale.Plot Name"="", "X Scale.Use Plot Name"=FALSE}}, "Load options (All)"={"Load plots?"=TRUE, "Load X-axis?"=TRUE, "Load Y-axes?"=TRUE, "Load General?"=TRUE}} ("Cluster"), Variant=w348) -> (data=w351:T32, error out=w350:errorcluster)  [unwired: 1 in]
            n198 = case shown="No Error" w350 {
              tunnel: w351 -> [w354 _]
              tunnel: w346 -> [w355 _]
              frame No Error {
                n199 = Unbundle By Name(w354) -> ("Plot config"=w353:T33, "Load options (All)"=w352:T31)
                n200 = call "Plot load reader V2.vi"("Load options (All)"=w352, "Plot config"=w353, "Refs"=w355) -> ()  [unwired: 8 in, 1 out]
              }
              frame Error {
              }
            }
          }
          frame "Clear Config" {
            w357 = 2  # # plots
            n201 = call "Plot init properties.vi"("# plots"=w357, "Refs"=w356) -> ()  [unwired: 8 in, 2 out]
          }
          frame "Set TimeToPlot" {
            n202 = Variant To Data(type=0.0, Variant=w360) -> (data=w363:dbl, error out=w362:errorcluster)  [unwired: 1 in]
            n203 = case shown="No Error" w362 {
              tunnel: w363 -> [w364 _]
              frame No Error {
                n204 = property on="Time to Plot" class="DigNum (strict)"("Val(Sgnl)"=w364) -> ()  [unwired: 2 in, 2 out]
              }
              frame Error {
              }
            }
          }
        }
      }
      event User Event {
        n205 = event-data() -> ("State"=w371:T44)  [unwired: 1 in]
        n206 = call <vilib>:"Is State Visible.vi"("Visibility"=w371) -> ("Visible"=w370:bool)  [unwired: 10 in]
        n207 = Bundle By Name(cluster=w369, "visible?"=w370) -> (w368:T14)
        n208 = call "calc timeout.vi"("init options"=w365, "Loop data in"=w368) -> ("Update?"=w366:bool, "timeout"=w367:i32)  [unwired: 8 in]
      }
      event User Event {
        w376 = TRUE
        n209 = event-data() -> ()  [unwired: 1 in, 5 out]
        n210 = Release Notifier(notifier=w375, force destroy? (F)=TRUE) -> ()  [unwired: 1 in, 3 out]
        n211 = call-dynamic "Callback - Shutdown.vi"("BluePlotHandle in"=w372) -> ()  [unwired: 9 in, 2 out]
        n212 = Unbundle By Name(w377) -> ("Meta LUT"=w382:refnum<data-value>, "TipPanel"=w373:refnum<class "TipPanelHandle.lvclass">)
        n213 = Delete Data Value Reference(data value reference=w382) -> ()  [unwired: 1 in, 2 out]
        n214 = call-poly <userlib>:"TipStrip API.vi"("TipPanelHandle"=w373) -> ()  [unwired: 10 in, 1 out]
        n215 = Unbundle By Name(w378) -> ("TitleCollapse"=w381:refnum<class "CollapsePanel.lvclass">, "keyboard"=w380:refnum<k1>)
        n216 = call-poly "POLY API.vi"("CollapsePanel in"=w381) -> ()  [unwired: 10 in, 1 out]
        n217 = call-poly <vilib>:"Close Input Device.vi"("device ID"=w380) -> ("error out"=w379:errorcluster)  [unwired: 9 in]
        n218 = call <vilib>:"Clear Errors.vi"("error in (no error)"=w379) -> ()  [unwired: 5 in, 2 out]
        n219 = property on="shutdown?" class="Bool (strict)"("Val(Sgnl)"=w376) -> ()  [unwired: 2 in, 2 out]
      }
      event Timeout {
        n220 = event-data() -> ()  [unwired: 1 in, 1 out]
        n221 = Unbundle By Name(w391) -> ("MouseDownState"=w390:T15)
        n222 = call "Plot Zoom Key Down Detect.vi"("Refs"=w386, "Loop data in"=w391) -> ("Loop data out"=w393:T14)  [unwired: 8 in, 1 out]
        n223 = call "Plot key focus color.vi"("Refs"=w386) -> ()  [unwired: 10 in, 1 out]
        n224 = case shown="\"Pan\", \"Zoom\"" w390 {
          tunnel: [TRUE ("enqueue update plot?") w397] -> w392
          tunnel: w389 -> [_ w396]
          tunnel: w391 -> [_ w395]
          frame Default {
          }
          frame "Pan", "Zoom" {
            n225 = call "Update plot calc.vi"("Init options"=w396, "Loop data"=w395) -> ("enqueue update plot?"=w397:bool)  [unwired: 9 in]
          }
        }
        n226 = call "ZoomPostEnd.vi"("Refs"=w386, "Loop data in"=w393) -> ("Loop data out"=w385:T14)  [unwired: 8 in, 1 out]
        n227 = case shown="True" w392 {
          tunnel: w385 -> [w398 w401]
          tunnel: [w398 w400] -> w384
          tunnel: w383 -> [_ w399]
          frame False {
          }
          frame True {
            n228 = call "Queue plot update.vi"("update plot notifier"=w399, "loop data in"=w401) -> ("loop data out"=w400:T14)  [unwired: 9 in]
          }
        }
        n229 = call "calc timeout.vi"("init options"=w389, "Loop data in"=w384) -> ("Update?"=w387:bool, "timeout"=w388:i32)  [unwired: 8 in]
      }
      event Value Change {
        n230 = event-data() -> ("NewVal.RightClickCache.slice"=w406:T2[], "NewVal.Numerics"=w403:dbl[])  [unwired: 1 in]
        n231 = Get Date/Time In Seconds() -> (seconds since 1Jan1904=w410:timestamp)
        n232 = To Double Precision Float(number=w410) -> (double precision float=w409:dbl)
        n233 = Bundle By Name(cluster=w407, "UpdateTime"=w409, "RightClickCache.slice"=w406) -> (w405:T14)
        n234 = call "Plot area resize.vi"("Refs"=w404) -> ("error out"=w402:errorcluster)  [unwired: 10 in]
        n235 = call "Plot update numeric array.vi"("Numerics"=w403, "refs"=w404) -> ()  [unwired: 9 in, 1 out]
        n236 = call "RightClickUpdate Wrapper.vi"("error in (no error)"=w402, "Refs"=w404, "Loop data in"=w405) -> ("Loop data out"=w408:T14)  [unwired: 7 in, 1 out]
      }
      event "Plot": Mouse Down? {
        n237 = event-data() -> ("CtlRef"=w419:refnum<vi>, "Coords"=w418:T12, "Button"=w417:u16, "PlatMods"=w414:T45)  [unwired: 1 in]
        n238 = Unbundle By Name(w425) -> ("MouseDownState"=w416:T15)
        n239 = call "Mouse Down Discard.vi"("Loopdata.MouseDownState"=w416, "PlatMods"=w414, "Button"=w417, "Coords"=w418, "plot reference"=w419) -> ("Discard?"=w412:bool, "Start new ToolTip?"=w415:bool, "command"=w411:T15)  [unwired: 4 in]
        n240 = case shown="True" w415 {
          tunnel: [w426 w435] -> w413
          tunnel: w424 -> [_ w434]
          tunnel: w411 -> [_ w433]
          tunnel: w414 -> [w426 w432]
          tunnel: [w427 w431] -> w420
          tunnel: w418 -> [_ w430]
          tunnel: w425 -> [w427 w429]
          frame False {
          }
          frame True {
            w428 = FALSE ("Shift")
            n241 = call "Mouse Down_ on PlotArea.vi"("Coords"=w430, "Loop data in"=w429, "PlatMods"=w432, "ScaleState"=w433, "Refs"=w434) -> ("Loop data out"=w431:T14)  [unwired: 5 in, 1 out]
            n242 = Bundle By Name(cluster=w432, "Shift"=w428, "Ctrl"=w428) -> (w435:T45)
          }
        }
        n243 = event-data("PlatMods"=w413, "Discard?"=w412) -> ()  [unwired: 1 in, 1 out]
        n244 = call "calc timeout.vi"("init options"=w423, "Loop data in"=w420) -> ("Update?"=w421:bool, "timeout"=w422:i32)  [unwired: 8 in]
      }
      event "Plot": Mouse Down {
        n245 = event-data() -> ("Coords"=w445:T12, "CtlRef"=w438:refnum<vi>)  [unwired: 1 in]
        n246 = call "Mouse Down on Markers.vi"("Coords"=w445, "Refs"=w439) -> ("target axis"=w446:T5, "Mouse down on axis marker?"=w447:bool, "ScaleRef"=w437:refnum<vi>)  [unwired: 6 in, 1 out]
        n247 = case shown="False" w447 {
          selector: w447 -> [_ w459]
          tunnel: w446 -> [_ w460]
          tunnel: w445 -> [w455 _]
          tunnel: [w454 w460] -> w442
          tunnel: [w453 w459] -> w444
          tunnel: w439 -> [w452 w458]
          tunnel: [w452 w458] -> w440
          tunnel: w437 -> [_ w457]
          tunnel: [_ w456] -> w436
          frame False {
            n248 = call "Mouse Down on Axis.vi"("Coords"=w455, "Refs"=w452) -> ("target axis"=w454:T5, "Mouse down on Axis?"=w453:bool)  [unwired: 6 in, 2 out]
          }
          frame True {
            n249 = call "Mouse Down on Marker MinMax.vi"("Scale ref"=w457) -> ("mouse down on marker min/max?"=w456:bool)  [unwired: 8 in, 2 out]
          }
        }
        n250 = case shown="True" w444 {
          tunnel: w440 -> [w449 w451]
          tunnel: [w449 w451] -> w443
          tunnel: w442 -> [_ w450]
          frame False {
          }
          frame True {
            n251 = call "Plot axis key focus set.vi"("target axis"=w450, "Refs"=w451) -> ()  [unwired: 9 in, 1 out]
          }
        }
        n252 = case shown="False" w436 {
          tunnel: w438 -> [_ w463]
          tunnel: w443 -> [w461 w462]
          tunnel: [w461 w462] -> w448
          frame True {
          }
          frame False {
            n253 = property class="XYGraph (strict)"(reference=w463, "Key Focus"=TRUE) -> ()  [unwired: 1 in, 2 out]
          }
        }
        n254 = call "Plot key focus color.vi"("Refs"=w448) -> ()  [unwired: 10 in, 1 out]
      }
      event "Plot": Mouse Move {
        n255 = event-data() -> ("Coords"=w471:T12)  [unwired: 1 in]
        n256 = call "Plot Zoom Key Down Detect.vi"("Refs"=w468, "Loop data in"=w470) -> ("Loop data out"=w469:T14)  [unwired: 8 in, 1 out]
        n257 = call "RightClickUpdate Wrapper.vi"("Coords (no change)"=w471, "Refs"=w468, "Loop data in"=w469) -> ("Loop data out"=w467:T14)  [unwired: 7 in, 1 out]
        n258 = call "Update plot calc.vi"("Init options"=w473, "Loop data"=w467) -> ("enqueue update plot?"=w472:bool)  [unwired: 9 in]
        n259 = case shown="True" w472 {
          tunnel: w467 -> [w474 w477]
          tunnel: [w474 w476] -> w466
          tunnel: w465 -> [_ w475]
          frame False {
          }
          frame True {
            n260 = call "Queue plot update.vi"("update plot notifier"=w475, "loop data in"=w477) -> ("loop data out"=w476:T14)  [unwired: 9 in]
          }
        }
      }
      event "Plot": Mouse Up {
        n261 = event-data() -> ()  [unwired: 1 in, 1 out]
        n262 = call "Mouse Up on Plot.vi"("Loop data in"=w485, "Refs"=w484) -> ("Loop data out"=w480:T14)  [unwired: 8 in, 1 out]
        n263 = call "Queue plot update.vi"("update plot notifier"=w478, "loop data in"=w480) -> ("loop data out"=w479:T14)  [unwired: 9 in]
        n264 = call "calc timeout.vi"("init options"=w481, "Loop data in"=w479) -> ("Update?"=w482:bool, "timeout"=w483:i32)  [unwired: 8 in]
      }
      event "Plot": Scale Range Change {
        n265 = event-data() -> ("ScaleRef"=w490:refnum<vi>, "NewRange"=w489:T21)  [unwired: 1 in]
        n266 = call "Plot scale range change.vi"("Loop data in"=w491, "NewRange"=w489, "ScaleRef"=w490, "Refs"=w492) -> ("Loop data out"=w488:T14)  [unwired: 6 in, 1 out]
        n267 = call "Queue plot update.vi"("update plot notifier"=w486, "loop data in"=w488) -> ("loop data out"=w487:T14)  [unwired: 9 in]
      }
      event "Plot": Key Down; "Plot": Key Repeat {
        n268 = event-data() -> ("CtlRef"=w501:refnum<vi>, "VKey"=w503:T46, "PlatMods"=w502:T45)  [unwired: 1 in]
        n269 = property class="XYGraph (strict)"(reference=w501) -> ("Key Focus"=w500:bool)  [unwired: 1 in, 2 out]
        n270 = case shown="True" w500 {
          tunnel: w505 -> [_ w511]
          tunnel: w504 -> [w510 w513]
          tunnel: [w510 w517] -> w495
          tunnel: w503 -> [_ w516]
          tunnel: w502 -> [_ w515]
          tunnel: [_ w514] -> w498
          frame False {
            # "user is editing the axis markers"
          }
          frame True {
            n271 = call "Plot Zoom Key Down Detect.vi"("Refs"=w511, "Loop data in"=w513) -> ("Loop data out"=w512:T14)  [unwired: 8 in, 1 out]
            n272 = call "Plot Key Down.vi"("Loop data in"=w512, "PlatMods"=w515, "VKey"=w516, "Refs"=w511) -> ("Update plot?"=w514:bool, "Loop data out"=w517:T14)  [unwired: 5 in, 1 out]
          }
        }
        n273 = call "Update plot calc.vi"("Init options"=w499, "Loop data"=w495) -> ("enqueue update plot?"=w497:bool)  [unwired: 9 in]
        n274 = Or(x=w497, y=w498) -> (x .or. y?=w496:bool)
        n275 = case shown="True" w496 {
          tunnel: w495 -> [w506 w509]
          tunnel: [w506 w508] -> w494
          tunnel: w493 -> [_ w507]
          frame False {
          }
          frame True {
            n276 = call "Queue plot update.vi"("update plot notifier"=w507, "loop data in"=w509) -> ("loop data out"=w508:T14)  [unwired: 9 in]
          }
        }
      }
      event "Plot": Key Up {
        n277 = event-data() -> ("CtlRef"=w526:refnum<vi>, "PlatMods"=w527:T45)  [unwired: 1 in, 1 out]
        n278 = property class="XYGraph (strict)"(reference=w526) -> ("Key Focus"=w525:bool)  [unwired: 1 in, 2 out]
        n279 = case shown="True" w525 {
          tunnel: w529 -> [_ w539]
          tunnel: w528 -> [w534 w538]
          tunnel: [w534 w537] -> w520
          tunnel: w527 -> [_ w535]
          tunnel: [_ w536] -> w523
          frame False {
            # "user is editing the axis markers"
          }
          frame True {
            n280 = call "Plot Key Up.vi"("Loop data in"=w538, "PlatMods"=w535, "Refs"=w539) -> ("Update plot?"=w536:bool, "Loop data out"=w537:T14)  [unwired: 6 in, 1 out]
          }
        }
        n281 = call "Update plot calc.vi"("Init options"=w524, "Loop data"=w520) -> ("enqueue update plot?"=w522:bool)  [unwired: 9 in]
        n282 = Or(x=w522, y=w523) -> (x .or. y?=w521:bool)
        n283 = case shown="True" w521 {
          tunnel: w520 -> [w530 w533]
          tunnel: [w530 w532] -> w519
          tunnel: w518 -> [_ w531]
          frame False {
          }
          frame True {
            n284 = call "Queue plot update.vi"("update plot notifier"=w531, "loop data in"=w533) -> ("loop data out"=w532:T14)  [unwired: 9 in]
          }
        }
      }
      event "Plot": Mouse Wheel {
        n285 = event-data() -> ("Coords"=w543:T12, "Delta"=w546:i32, "PlatMods"=w545:T45)  [unwired: 1 in]
        n286 = call "Plot Mouse Wheel.vi"("PlatMods"=w545, "Loop data in"=w547, "Delta"=w546, "Coords"=w543, "Refs"=w548) -> ("Update plot?"=w544:bool, "Loop data out"=w541:T14)  [unwired: 4 in, 1 out]
        n287 = case shown="True" w544 {
          tunnel: [w549 w552] -> w542
          tunnel: w541 -> [w549 w551]
          tunnel: w540 -> [_ w550]
          frame False {
          }
          frame True {
            n288 = call "Queue plot update.vi"("update plot notifier"=w550, "loop data in"=w551) -> ("loop data out"=w552:T14)  [unwired: 9 in]
          }
        }
      }
      event "Info": Value Change {
        n289 = event-data() -> ("NewVal"=w555:bool)  [unwired: 1 in]
        n290 = Unbundle By Name(w554) -> ("TipPanel"=w553:refnum<class "TipPanelHandle.lvclass">)
        n291 = Unbundle By Name(w554) -> ("Plot"=w557:refnum<vi>)
        n292 = property class="XYGraph (strict)"(reference=w557, "Key Focus"=TRUE) -> ()  [unwired: 1 in, 2 out]
        n293 = call "Info button.vi"("TipPanelHandle"=w553, "Info"=w555) -> ()  [unwired: 10 in]
      }
      event "Info": Mouse Move {
        n294 = event-data() -> ()  [unwired: 1 in, 1 out]
        n295 = Unbundle By Name(w560) -> ("TipPanel"=w559:refnum<class "TipPanelHandle.lvclass">)
        n296 = call "Info button.vi"("TipPanelHandle"=w559, "Info"="Info") -> ()  [unwired: 10 in]
      }
      event "Info": Mouse Leave {
        n297 = event-data() -> ("CtlRef"=w566:refnum<vi>)  [unwired: 1 in, 3 out]
        n298 = property class="Bool (strict)"(reference=w566, "Value"=FALSE) -> ()  [unwired: 1 in, 2 out]
        n299 = Unbundle By Name(w564) -> ("TipPanel"=w563:refnum<class "TipPanelHandle.lvclass">)
        n300 = call <userlib>:"CMD - hide.vi"("TipPanelHandle"=w563) -> ()  [unwired: 9 in, 2 out]
      }
      event "max": Value Change {
        n301 = event-data() -> ("NewVal"=w572:bool)  [unwired: 1 in]
        n302 = control-ref of="max"() -> (w573:refnum<vi>)
        n303 = Unbundle By Name(w579) -> ("Plot"=w582:refnum<vi>)
        n304 = property class="RocketPlotHandle.lvclass"(reference=w569) -> ("callback UE"=w568:refnum<user-event>)  [unwired: 1 in, 2 out]
        n305 = property class="XYGraph (strict)"(reference=w582, "Key Focus"=TRUE) -> ()  [unwired: 1 in, 2 out]
        n306 = Bundle By Name(cluster=T38 {"Maximize?"=FALSE, "max button"=refnum} ("Cluster"), "Maximize?"=w572, "max button"=w573) -> (w574:T38)
        n307 = call <vilib>:"Get SubPanel.vi"("Panel in"=w570) -> ("SubPanel"=w571:refnum<vi>)  [unwired: 8 in, 2 out]
        n308 = Bundle By Name(cluster=T29 {"Type"=enum."Maximize", "data"=variant(string ""), "owning subpanel"=refnum} ("event data"), "Type"=callback_type."Maximize", "owning subpanel"=w571, "data"=w574) -> (w577:T29)
        n309 = Generate User Event(user event=w568, event data cluster=w577) -> ()  [unwired: 2 in, 2 out]
      }
      event "max": Mouse Move {
        n310 = event-data() -> ()  [unwired: 1 in, 1 out]
        n311 = case shown="True" "max" {
          tunnel: ["Click to maximize  <F11>" ("String") "Click to restore  <F11>" ("String")] -> w585
          frame False {
          }
          frame True {
          }
        }
        n312 = Unbundle By Name(w584) -> ("TipPanel"=w583:refnum<class "TipPanelHandle.lvclass">)
        n313 = call "new cell.vi"("String"=w585) -> ("cell"=w588:T42)  [unwired: 10 in]
        n314 = Build Array(w588) -> (w589:T42[])
        n315 = Build Array(w589) -> (w587:T42[][])
        n316 = call "New TipTable.vi"("show.cells"=w587) -> ("TipTablePanel out"=w586:refnum<class "TipTablePanel.lvclass">)  [unwired: 9 in, 1 out]
        n317 = call-poly <userlib>:"TipStrip API.vi"("TipPanel"=w586, "TipPanelHandle"=w583) -> ()  [unwired: 8 in, 2 out]
      }
      event "max": Mouse Leave {
        n318 = event-data() -> ()  [unwired: 1 in, 4 out]
        n319 = Unbundle By Name(w595) -> ("TipPanel"=w594:refnum<class "TipPanelHandle.lvclass">)
        n320 = call <userlib>:"CMD - hide.vi"("TipPanelHandle"=w594) -> ()  [unwired: 9 in, 2 out]
      }
      event "x-axis not time?": Value Change {
        w611 = u8 2 ("Scale Fit")
        n321 = event-data() -> ("NewVal"=w603:bool)  [unwired: 1 in]
        n322 = Unbundle By Name(w610) -> ("Plot"=w606:refnum<vi>, "Left Scale"=w607:refnum<vi>, "Right Scale"=w608:refnum<vi>, "TimeZone"=w613:refnum<vi>, "Meta LUT"=w617:refnum<data-value>, "X Scale"=w618:refnum<vi>, "spoof"=w602:refnum<vi>, "X Scale.Plot Name"=w628:refnum<vi>)
        n323 = property class="Str"(reference=w628, "Visible"=w603) -> ()  [unwired: 1 in, 2 out]
        n324 = Select(t="%#_g" ("Format String"), s=w603, f="%<%H:%M:%S>T" ("Format String")) -> (s? t:f=w614:string)
        n325 = Select(t="X Axis" ("Format String"), s=w603, f="Time (s)" ("Format String")) -> (s? t:f=w600:string)
        n326 = call "Plot Load maker V2 - scaleread grid colors.vi"("Scale reference"=w618, "Meta LUT"=w617) -> ("error out"=w623:errorcluster, "Scale LUT meta"=w624:T47, "Scale reference"=w625:refnum<vi>, "Meta LUT"=w626:refnum<data-value>)  [unwired: 6 in]
        n327 = Bundle By Name(cluster=w624, "Format String"=w614) -> (w627:T47)
        n328 = property class="Enum (strict)"(reference=w613) -> ("Value"=w619:T49)  [unwired: 1 in, 2 out]
        n329 = call "Plot index to active axis.vi"("Plot"=w602) -> ("Scale reference"=w601:refnum<vi>)  [unwired: 8 in, 2 out]
        n330 = call "Plot Load maker V2 - scalewrite grid colors.vi"("error in (no error)"=w623, "Meta"=w627, "Scale reference"=w625, "Meta LUT"=w626) -> ("error out"=w622:errorcluster, "Scale reference"=w620:refnum<vi>, "Meta LUT"=w621:refnum<data-value>)  [unwired: 5 in]
        n331 = call "Plot axes format string.vi"("TimeZone"=w619, "error in (no error)"=w622, "Scale reference"=w620, "Meta LUT"=w621) -> ("Scale reference"=w609:refnum<vi>)  [unwired: 6 in, 1 out]
        n332 = property class="XYGraph (strict)"(reference=w606, "ActPaletteTool"=0 ("Palette:Active Tool")) -> ()  [unwired: 1 in, 2 out]
        n333 = property class="GrphScl"(reference=w607, "ScaleFit"=w611) -> ()  [unwired: 1 in, 2 out]
        n334 = property class="GrphScl"(reference=w608, "ScaleFit"=w611) -> ()  [unwired: 1 in, 2 out]
        n335 = property class="GrphScl"(reference=w609, "ScaleFit"=w611, "NameLbl.Text"=w600) -> ()  [unwired: 1 in, 2 out]
        n336 = property class="GraphScale"(reference=w601, "NameLbl.Text"=w600) -> ()  [unwired: 1 in, 2 out]
        n337 = call "Queue plot update.vi"("update plot notifier"=w597, "loop data in"=w599) -> ("loop data out"=w598:T14)  [unwired: 9 in]
      }
      event "x-axis name": Mouse Down {
        n338 = event-data() -> ("Button"=w629:u16)  [unwired: 1 in]
        n339 = case shown="1" w629 {
          tunnel: w631 -> [_ w651]
          tunnel: w630 -> [_ w646]
          frame Default {
          }
          frame 1 {
            n340 = call-dynamic "Callback - Get Plottable Names.vi"("BluePlotHandle in"=w651) -> ("Plottable Names"=w647:string[])  [unwired: 8 in, 2 out]
            n341 = Unbundle By Name(w646) -> ("X Scale.Plot Name"=w644:refnum<vi>, "tab ref"=w639:refnum<vi>, "LegendPane"=w637:refnum<vi>, "VI"=w636:refnum<vi>)
            n342 = property on="Property Node" class="Str"(reference=w644) -> (reference out=w640:refnum<vi>, "Value"=w643:string)  [unwired: 1 in, 1 out]
            n343 = property on="Property Node" class="TabCtl (strict)"(reference=w639) -> ("Position"=w638:T50)  [unwired: 1 in, 2 out]
            n344 = call "PaneCoordsToScreenCoords.vi"("VI"=w636, "Origin Pane"=w637, "Owning Pane"=w637, "Pane Coordinates"=w638) -> ("Screen Coords"=w635:T25)  [unwired: 6 in, 1 out]
            n345 = Add(x=T25 {"Horizontal"=19, "Vertical"=94}, y=w635) -> (x+y=w633:T25)
            n346 = Bundle By Name(cluster=T39 {"Screen Coordinates"={"Horizontal"=0, "Vertical"=0}, "Width"=0, "max rows"=8, "List"=[], "init value"=""} ("input"), "Width"=u32 500, "max rows"=30, "List"=w647, "init value"=w643, "Screen Coordinates"=w633) -> (w645:T39)
            n347 = call "Autocomplete popup.vi"("input"=w645) -> ("Accept?"=w642:bool, "String"=w641:string)  [unwired: 8 in, 1 out]
            n348 = case shown="True" w642 {
              tunnel: w641 -> [_ w653]
              tunnel: w640 -> [_ w652]
              frame False {
              }
              frame True {
                n349 = property on="Property Node" class="Str"(reference=w652, "Value"=w653) -> ()  [unwired: 1 in, 2 out]
              }
            }
          }
        }
      }
      event "top array": Mouse Down {
        n350 = event-data() -> ("Button"=w656:u16)  [unwired: 1 in]
        n351 = case shown="1" w656 {
          tunnel: w657 -> [_ w659]
          tunnel: w654 -> [_ w658]
          frame Default {
          }
          frame 1 {
            # "left click"
            n352 = Unbundle By Name(w659) -> ("top array"=w664:refnum<vi>, "TopArray.PID"=w663:refnum<vi>)
            n353 = call "Array Point to RowCol V3.vi"("PID"=w663, "top array"=w664) -> ("Flatline?"=w660:bool, "Index"=w661:i32, "PID key focus?"=w662:bool)  [unwired: 6 in, 1 out]
            n354 = case shown="True" w662 {
              tunnel: w661 -> [_ w667]
              tunnel: w660 -> [_ w668]
              tunnel: w659 -> [_ w666]
              tunnel: w658 -> [_ w665]
              frame False {
              }
              frame True {
                n355 = call "activate autocomplete v2.vi"("BluePlotHandle in"=w665, "Refs"=w666, "Flatline?"=w668, "Index"=w667) -> ()  [unwired: 7 in, 1 out]
              }
            }
          }
        }
      }
      event "top array": Value Change {
        n356 = event-data() -> ("NewVal"=w671:T8[], "OldVal"=w672:T8[])  [unwired: 1 in]
        n357 = call "Plot TopArray ValueChange.vi"("OldVal"=w672, "NewVal"=w671, "Refs"=w670) -> ()  [unwired: 8 in, 1 out]
      }
      event "Add row": Value Change {
        n358 = event-data() -> ()  [unwired: 1 in, 1 out]
        n359 = call "Plot add row.vi"("Refs"=w674) -> ("error out"=w675:errorcluster)  [unwired: 10 in]
        n360 = call "Plot resize vertical.vi"("error in (no error)"=w675, "Refs"=w674) -> ()  [unwired: 7 in, 3 out]
      }
    }
    n361 = call "plot Timeout Helper.vi"("new timeout?"=w95, "new timeout mS"=w94, "Timeout"=w96) -> ("Timeout"=w97:i32)  [unwired: 8 in]
  }
  n362 = while {
    tunnel: [w680] -> w10
    tunnel: w9 -> [w682]
    tunnel: w8 -> [w681]
    tunnel: w5 -> [w678]
    tunnel: w6 -> [w679]
    stop <- w680 stop-if-true
    # "Settings UI in separate loop so that user can watch changes in real time"
    n363 = Wait on Notification(notifier=w679, error in (no error)=w678) -> (notification=w676:T10, error out=w677:errorcluster)  [unwired: 2 in, 2 out]
    n364 = case shown="No Error" w677 {
      tunnel: w682 -> [w702 _]
      tunnel: w681 -> [w701 _]
      tunnel: [_ TRUE] -> w680
      tunnel: w676 -> [w687 _]
      frame No Error {
        n365 = local read "Time to Plot"() -> (w691:dbl)
        n366 = local read "top array"() -> (w700:T8[])
        n367 = call "has changed boolen - init first call.vi"("Boolean in"="Erase Plot") -> ("has changed?"=w696:bool, "Boolean out"=w697:bool)  [unwired: 9 in]
        n368 = call "has changed dbl first call.vi"("Numeric"=w691) -> ("has changed?"=w694:bool, "Numeric (dup)"=w699:dbl)  [unwired: 9 in]
        n369 = Compound Arithmetic op=AND(w697, w696) -> (w698:bool)
        n370 = Compound Arithmetic op=AND(invert w697, w696) -> (w695:bool)
        n371 = Or(x=w695, y=w694) -> (x .or. y?=w693:bool)
        n372 = call "Get Oldest Time to Plot.vi"("reset? [F]"=w693, "History Length (s)"=w699, "Clear Plot [F]"=w698) -> ("clear button active?"=w692:bool, "Oldest Time to Plot"=w689:u64)  [unwired: 7 in]
        n373 = call "Plot Update.vi"("BluePlotHandle"=w702, "update plot"=w687, "top array"=w700, "Oldest Time to Plot (autoscaled)"=w689, "refs"=w701) -> ("Numerics"=w684:dbl[], "Plot"=w688:cluster{dbl[], "Data":dbl[]}[], "RightClickCache.slice"=w685:T2[])  [unwired: 3 in, 1 out]
        n374 = Bundle By Name(cluster=T1 {"Numerics"=[], "RightClickCache.slice"=[]} ("Cluster"), "RightClickCache.slice"=w685, "Numerics"=w684) -> (w683:T1)
        n375 = property on="Plot Updated" class="Clust (strict)"("Val(Sgnl)"=w683) -> ()  [unwired: 2 in, 2 out]
        n376 = local write "Erase Plot"(w692) -> ()
        n377 = local write "Plot"(w688) -> ()
      }
      frame Error {
      }
    }
  }
  n378 = while {
    tunnel: w8 -> [w705]
    tunnel: [w704] -> w12
    stop <- w704 stop-if-true
    # "Settings UI in separate loop so that user can watch changes in real time"
    n379 = event shown="[0] \"Open Settings (spoof)\", \"Open Settings\": Value Change" {
      selector: _ -> [_ _]
      dyn-events: _ -> [_ _]
      timeout: _ -> [_ _]
      tunnel: w705 -> [w706 _]
      tunnel: [_ TRUE] -> w704
      event "Open Settings (spoof)", "Open Settings": Value Change {
        n380 = event-data() -> ()  [unwired: 1 in, 1 out]
        n381 = call "Plot Scales GUI V2.vi"("Refs"=w706) -> ()  [unwired: 10 in, 1 out]
      }
      event "shutdown?": Value Change {
        n382 = event-data() -> ()  [unwired: 1 in, 1 out]
      }
    }
  }
  n383 = flat-sequence {
    tunnel: w45 -> [w710]
    tunnel: w2 -> [w708]
    tunnel: w12 -> [_]
    tunnel: w10 -> [_]
    frame #0 {
      # "shutdown"
      n384 = Unregister For Events(event registration refnum=w710) -> ()  [unwired: 1 in, 1 out]
      n385 = call <vilib>:"Set Running.vi"("Running"=FALSE, "Panel in"=w708) -> ()  [unwired: 8 in, 2 out]
    }
  }
